vi "运维调试_总氮.vi"() -> ()   [LabVIEW 2016, in "斯坦道总氮.lvlib"]
uses:
  <vilib>/Utility/miscctls.llb/LVPointTypeDef.ctl
  <vilib>/Utility/config.llb/NI_LVConfig.lvlib
  <vilib>/ptbypt/NI_PtbyPt.lvlib
panel:
  in  "远程标样校准":enum16{"标液1", "标液2", "标液3", "标液4"}(ring)
  in  "远程校准量程":enum16{"低量程", "高量程"}(ring)
  out "固件版本号":string
  in  "定时设置":cluster{"启动":bool, "控制命令":T1, "测量参数":T2}(xcontrol)
  out "单位:":T3(ring)
  out "模块版本号":string
  in  "校准按钮":T4
  out "运行状态":T5 {"数据时间:" format="%<%y/%m/%d %H:%M:%S>T"; "仪器时间:" format="%<%y/%m/%d %H:%M:%S>T"}
  out "一级权限":bool
  out "二级权限":bool
  out "输入密码":u32
  out "布尔":bool
  in  "流程固件":bool
  in  "仪器参数设置":bool
  in  "量程参数读取":T6
  in  "模块启用":bool
  in  "串口设置":bool
  in  "公式一键写入":bool
  in  "流程路径":path=path "C:/Users/STD/Documents/斯坦道流程文件/流程.xml"
  in  "曲线模型":cluster{"X^2":dbl, "X":dbl, "B":dbl, "r^2":dbl}(xcontrol)
  out "字符串":string
  in  "质控参数设置":bool
  out "温度2":sgl
  out "温度1":sgl
  out "ADC":sgl
  in  "数组":string[](array[string])
  in  "量程切换阈值写入":bool
  in  "量程切换阈值读取":bool
  in  "参数下拉列表":enum16{"总磷", "总氮"}(ring)=enum."总氮"
  in  "量程下拉列表":enum16{"低量程", "高量程"}(ring)
  in  "测量模式下拉列表":enum16{"水样测量", "零点核查", "跨度核查", "标样核查", "加标回收"}(ring)
  in  "公式":cluster{"X^2":dbl, "X":dbl, "b":dbl}
  in  "写公式":bool
  in  "读公式":bool
  in  "返回":bool
  in  "设置":bool
  out "集成报警信息":string
  in  "停止":bool
  in  "手动启动":bool
  in  "单步测试":bool
  out "F3":sgl format="%#.6f"
  out "F2":sgl format="%#.6f"
  out "F1":sgl format="%#.6f"
  out "F0":sgl format="%#.6f"
  out "多列列表框":i32(listbox)
  # "参数设置"
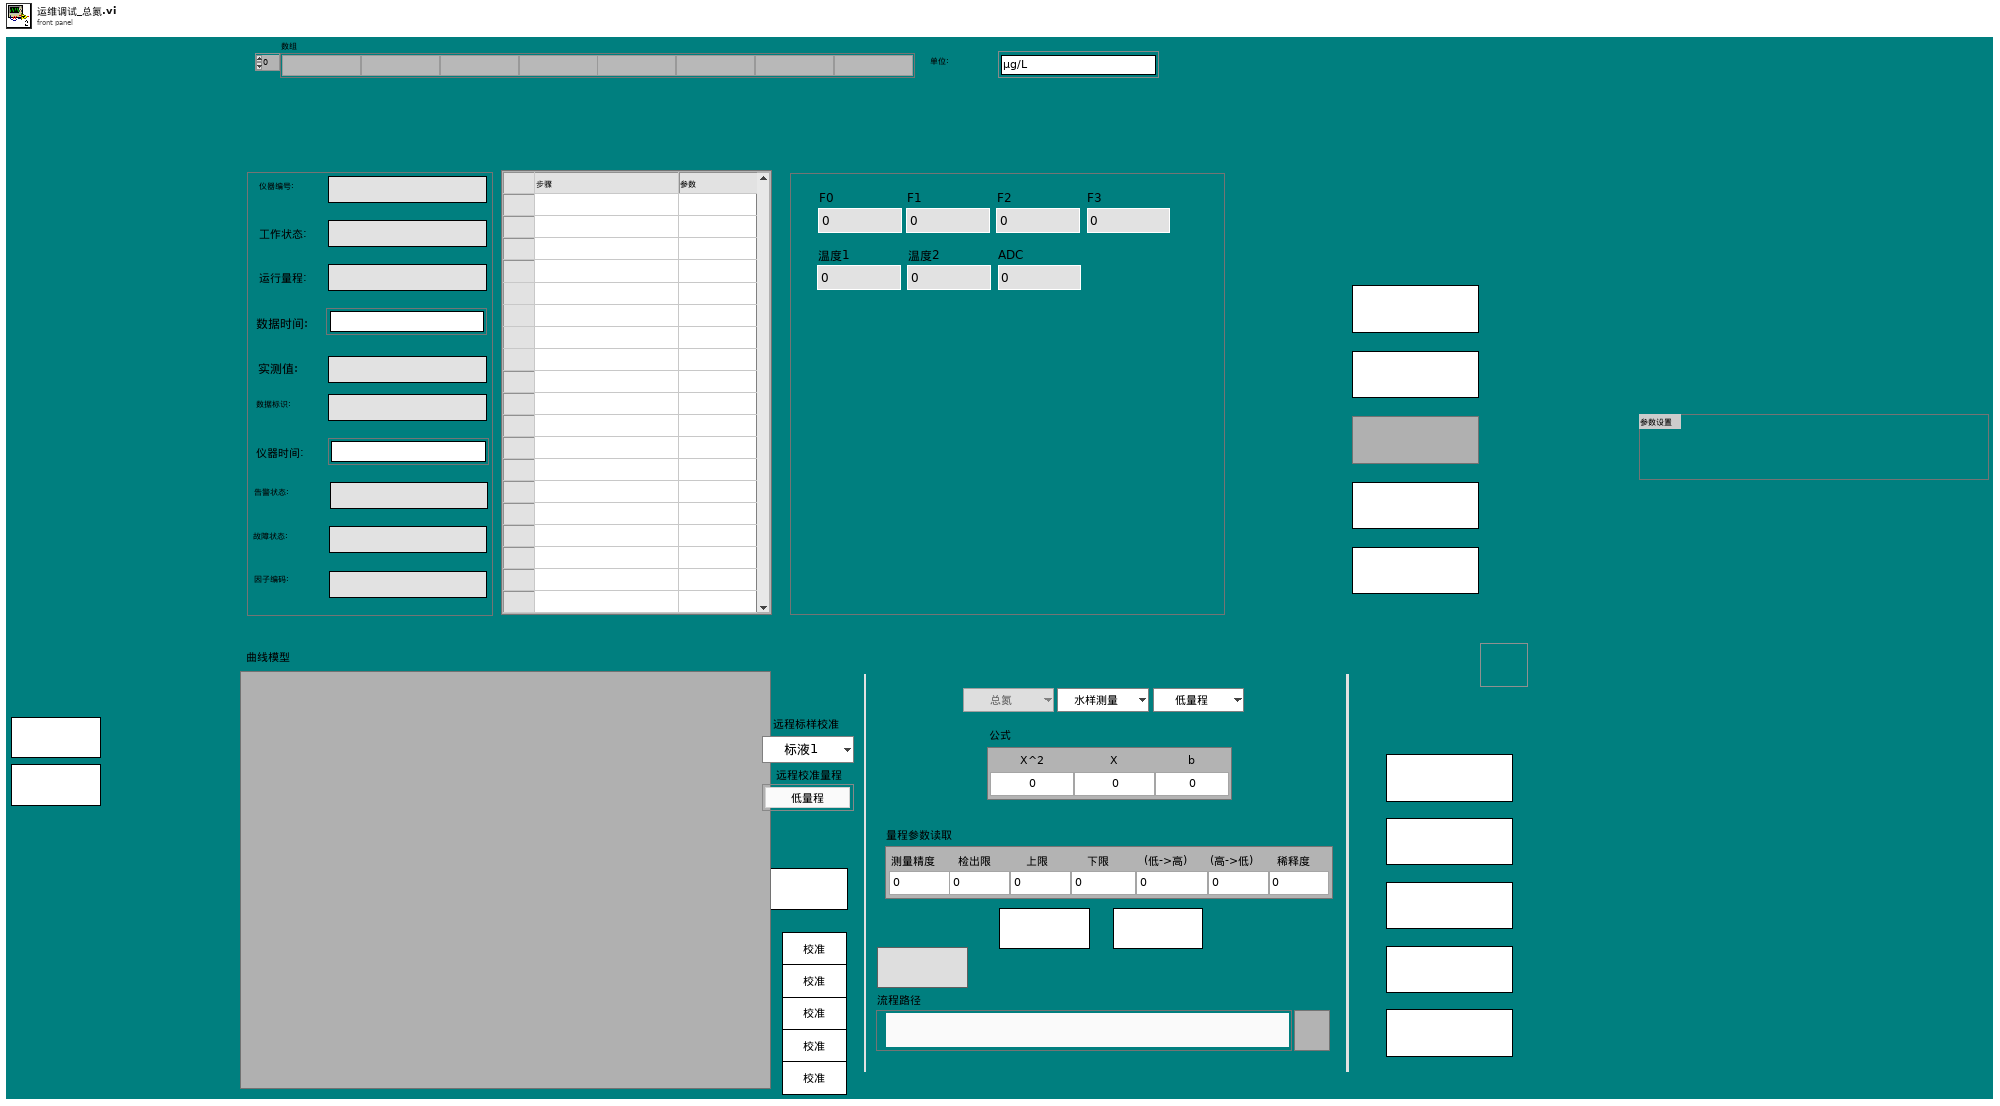
[diagram p1: front panel]
types:
  T1 = typedef "定时设置.xctl/国标控制命令.ctl" = enum16{"启动测量", "标样核查", "零点核查", "跨度核查", "空白测试", "平行样测试", "加标回收", "空白校准", "标样校准", "初始化（清洗）", "停止测试", "仪器重启", "校时", "模式设置", "测量间隔设置"}
  T2 = typedef "定时设置.xctl/测量参数.ctl" = u16
  T3 = enum16{"μg/L", "mg/L", "ppm", "mg/m3", "cm", "ppb", "μg/m3", "%", "nmol/mol", "μmol/mol", "MPN/L", "MPN/100ml", "ng/m3", "NTU", "无量纲", "mS/cm", "μS/cm", "℃", "mV", "cells/mL"}
  T4 = cluster{"校准1":bool, "校准2":bool, "校准3":bool, "校准4":bool, "校准5":bool}
  T5 = cluster{"仪器编号:":string, "工作状态:":string, "运行量程: ":string, "数据时间:":timestamp, "实测值:":string, "数据标识: ":string, "仪器时间:":timestamp, "告警状态: ":string, "故障状态:  ":string, "因子编码:":string}
  T6 = cluster{"测量精度":dbl, "检出限":dbl, "上限":dbl, "下限":dbl, "(低->高)":dbl, "(高->低)":dbl, "稀释度":dbl}
  T7 = typedef "LVPointTypeDef.ctl" = cluster{"Horizontal":i16, "Vertical":i16}
  T8 = cluster{"因子编码":u32, "单位":u16, "标样参考值":sgl, "水样数据时间":timestamp, "水样实测值":sgl, "水样数据标识":string, "标样数据时间":timestamp, "标样实测值":sgl, "标样数据标识":string, "空白数据时间":timestamp, "空白实测值":sgl, "空白数据标识":string, "零点核查数据时间":timestamp, "零点核查实测值":sgl, "零点核查数据标识":string, "跨度核查数据时间":timestamp, "跨度核查实测值":sgl, "跨度核查数据标识":string, "加标回收数据时间":timestamp, "加标回收实测值":sgl, "加标回收数据标识":string, "平行样数据时间":timestamp, "平行样实测值":sgl, "平行样数据标识":string, "F0":sgl, "F1":sgl, "F2":sgl, "F3":sgl, "F4":sgl, "F5":sgl, "F6":sgl, "F7":sgl, "温度":sgl, "湿度":sgl, "X值":sgl, "fidrange":u16}
  T9 = cluster{"系统时间":timestamp, "工作状态":enum16{"空闲", "水样测试", "标样核查", "零点核查", "跨度核查", "空白测试", "平行样测试", "加标回收", "空白校准", "标样校准", "初始化（清洗）"}, "测量模式":enum16{"待机", "连续模式", "周期模式", "定点模式", "受控模式", "手动模式"}, "告警代码":u16, "故障代码":u16, "日志代码":u16, "软件版本":u16, "F0":sgl, "F1":sgl, "F2":sgl, "F3":sgl, "T":sgl, "H":sgl, "id":u16, "flowid":u16, "量程":u16, "总磷控温温度1":sgl, "营养盐控温温度2":sgl, "ADC":sgl}
  T10 = enum16{"空闲", "水样测试", "标样核查", "零点核查", "跨度核查", "空白测试", "平行样测试", "加标回收", "空白校准", "标样校准", "初始化（清洗）"}
  T11 = cluster{"Major":u16, "Minor":u16, "Fix":u16, "Build":u16}
  T12 = typedef "NI_LVConfig.lvlib/Config Data RefNum.ctl" = refnum<k1>
  T13 = cluster{"时间源选择":enum16{"系统时间源", "仪器时间源"}, "外部时间源":timestamp}
  T14 = enum32{"Bad", "Idle", "Run top level", "Running"}
  T15 = enum8{"Enabled", "Disabled", "Disabled and Grayed Out"}
  T16 = cluster{"运行模式":enum16{"维护模式", "常规模式", "应急模式", "质控模式"}, "质控频次":enum16{"关闭", "每天", "星期一", "星期二", "星期三", "星期四", "星期五", "星期六", "星期日"}, "空白核查时间":u16, "跨度核查时间":u16, "24H周期设置":bool[]}
  T17 = cluster{"时间标识":timestamp, "设备":string, "日志信息":string, "备注":string}
  T18 = cluster{"参数":string, "报警内容":string, "报警分析":string}
  T19 = cluster{"启动模式":enum16{"跨度核查", "水样测量", "空白核查", "标样核查", "加标回收"}, "启动参数":u16, "量程":enum16{"低量程", "高量程"}}
  T20 = cluster{"时间标识":timestamp, "设备":string, "日志信息":string, "流程参数":string}
  T21 = typedef "LVRowAndColumnUnsignedTypeDef.ctl" = cluster{"Row":u32, "Column":u32}
  T22 = cluster{"参数下拉列表":enum16{"总磷", "总氮"}, "测量模式下拉列表":enum16{"水样测量", "零点核查", "跨度核查", "标样核查", "加标回收"}, "量程下拉列表":enum16{"低量程", "高量程"}}
  T23 = cluster{"站号":u16, "量程切换":enum32{"H", "L", "AUTO"}, "控制命令":enum16{"启动测量", "标样核查", "零点核查", "跨度核查", "空白测试", "平行样测试", "加标回收", "空白校准", "标样校准", "初始化（清洗）", "停止测试", "仪器重启", "校时", "模式设置", "测量间隔设置"}, "模式设置":enum16{"待机", "连续模式", "周期模式", "定点模式", "受控模式", "手动模式"}, "测量间隔":u16}
  T24 = cluster{"水样测试量程模式":enum16{"H", "L", "AUTO"}, "空白核查量程模式":enum16{"H", "L", "AUTO"}, "跨度核查量程模式":enum16{"H", "L", "AUTO"}, "加标回收量程模式":enum16{"H", "L", "AUTO"}}
  T25 = cluster{"跨度值":dbl, "零点标准液浓度":dbl, "跨度标准液浓度":dbl, "标准液标准浓度":dbl}
  T26 = cluster{"确定":bool, "跨度值":dbl, "零点标准液浓度":dbl, "跨度标准液浓度":dbl, "标准液标准浓度":dbl}
  T27 = cluster{"测量量程":dbl, "测量精度":dbl, "测量间隔":dbl, "消解温度":dbl, "消解时长":dbl, "空白校准时间":timestamp, "曲线截距":dbl, "曲线斜率":dbl, "测量检出限":dbl, "测量信号值":dbl, "线性相关系数":dbl, "二次多项式系数":dbl, "标样校准时间":timestamp, "稀释倍数":dbl, "三项式系数":dbl, "空白标定系数":dbl, "量程系数":dbl, "F0/ORPA":dbl, "F1/ORPB":dbl, "F2/ORPK":dbl, "F3":dbl, "F4":dbl, "F5":dbl, "F6":dbl, "F7":dbl, "X0/滴定数":dbl, "量程":dbl}
  T28 = cluster{"确定":bool, "测量量程":dbl, "测量精度":dbl, "测量间隔":dbl, "消解温度":dbl, "消解时长":dbl, "空白校准时间":timestamp, "曲线截距":dbl, "曲线斜率":dbl, "测量检出限":dbl, "测量信号值":dbl, "线性相关系数":dbl, "二次多项式系数":dbl, "标样校准时间":timestamp, "稀释倍数":dbl, "三项式系数":dbl, "空白标定系数":dbl, "量程系数":dbl, "F0/ORPA":dbl, "F1/ORPB":dbl, "F2/ORPK":dbl, "F3":dbl, "F4":dbl, "F5":dbl, "F6":dbl, "F7":dbl, "X0/滴定数":dbl, "量程":dbl}
  T29 = cluster{"标液浓度1":dbl, "标液浓度2":dbl, "标液浓度3":dbl, "标液浓度4":dbl, "标液浓度5":dbl}
  T30 = cluster{"测量精度":u16, "检出限":dbl, "上限":dbl, "下限":dbl, "阈值（低->高）":dbl, "阈值（高->低）":dbl, "稀释度":dbl}
  T31 = enum16{"Left Button", "Center Button", "Right Button", "Window Close"}
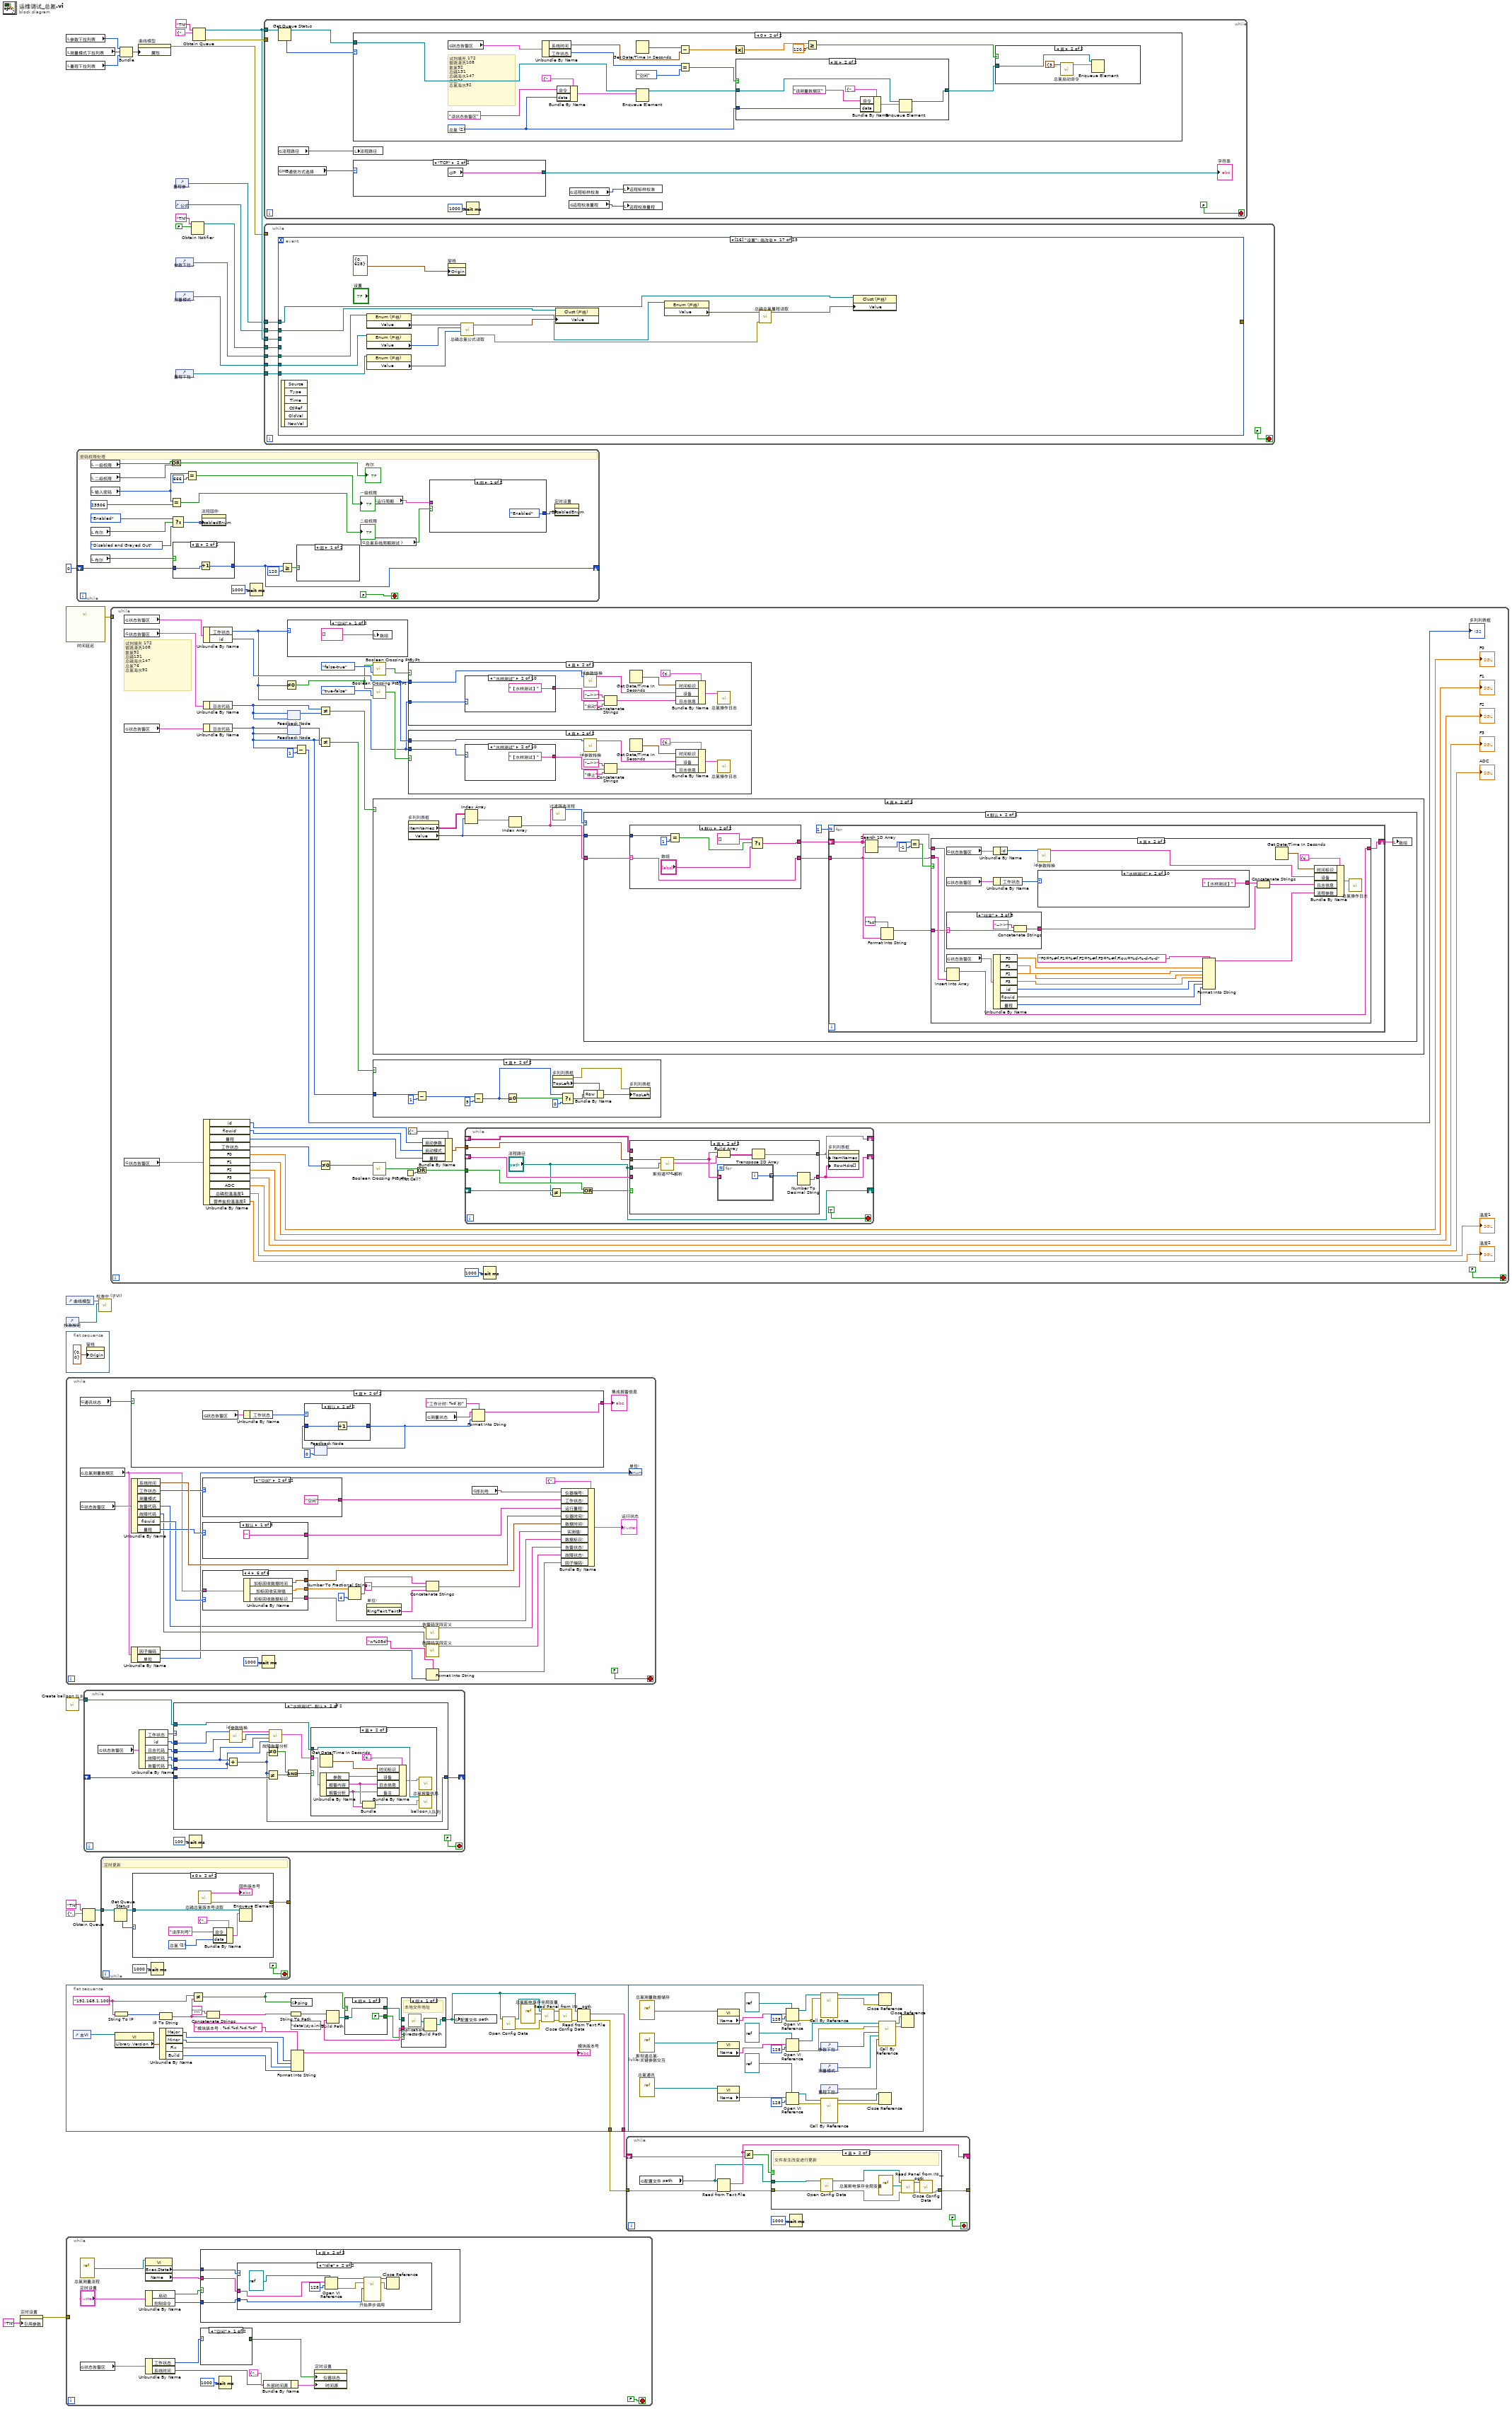
[diagram p0: block diagram]
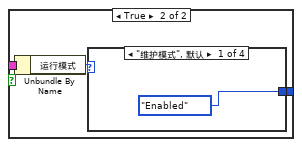
[diagram p5: hidden frame]
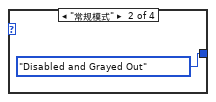
[diagram p6: hidden frame]
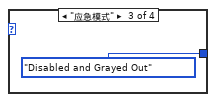
[diagram p7: hidden frame]
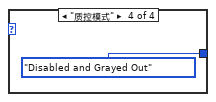
[diagram p8: hidden frame]
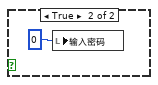
[diagram p9: hidden frame]
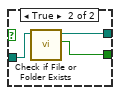
[diagram p11: hidden frame]
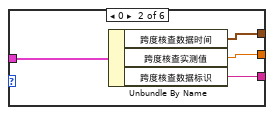
[diagram p15: hidden frame]
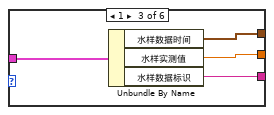
[diagram p16: hidden frame]
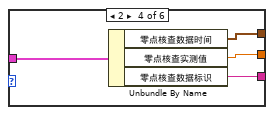
[diagram p17: hidden frame]
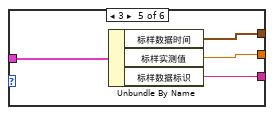
[diagram p18: hidden frame]
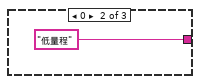
[diagram p19: hidden frame]
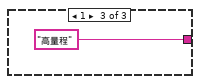
[diagram p20: hidden frame]
diagram:
  n1 = property on="定时设置" class="定时设置 (严格)"("引用参数"="TN") -> (error out=w1:errorcluster)  [unwired: 2 in, 1 out]
  n2 = local read "参数下拉列表"() -> (w12:enum16{"总磷", "总氮"})
  n3 = local read "测量模式下拉列表"() -> (w11:enum16{"水样测量", "零点核查", "跨度核查", "标样核查", "加标回收"})
  n4 = local read "量程下拉列表"() -> (w10:enum16{"低量程", "高量程"})
  n5 = call "时间延迟"() -> ("error out"=w21:errorcluster)  [unwired: 11 in]
  n6 = control-ref of="曲线模型"() -> (w6:refnum<vi>)
  n7 = control-ref of="校准按钮"() -> (w5:refnum<vi>)
  n8 = flat-sequence {
    frame #0 {
      n9 = property on="窗格" class="Pane"("Origin"=T7 {"Horizontal"=0, "Vertical"=0} ("原点")) -> ()  [unwired: 2 in, 2 out]
    }
  }
  n10 = while {
    stop <- FALSE stop-if-true
    n11 = global read "VAR总氮全局变量.vi" "通讯状态"() -> (w59:bool)
    n12 = global read "VAR总氮全局变量.vi" "总氮测量数据区"() -> (w48:T8)
    n13 = global read "VAR总氮全局变量.vi" "状态告警区"() -> (w51:T9)
    n14 = case shown="真" w59 {
      tunnel: ["通讯异常" ("集成报警信息") w102] -> w58
      frame False {
      }
      frame True {
        n15 = global read "VAR总氮全局变量.vi" "状态告警区"() -> (w108:T9)
        n16 = Unbundle By Name(w108) -> ("工作状态"=w107:T10)
        n17 = feedback #1(0) -> (w105:i32)
        n18 = case shown="默认" w107 {
          tunnel: w105 -> [_ w110]
          tunnel: [_ w109] -> w103
          frame "空闲" {
          }
          frame Default {
            n19 = Increment(x=w110) -> (x+1=w109:i32)
          }
        }
        n20 = feedback-in #1(w103) -> ()
        n21 = global read "VAR总氮全局变量.vi" "测量状态"() -> (w101:string)
        n22 = Format Into String(format string="工作计时: %d 秒" ("格式字符串"), initial string=w101, w103) -> (resulting string=w102:string)  [unwired: 1 in, 1 out]
      }
    }
    "集成报警信息" <- w58
    n23 = Unbundle By Name(w51) -> ("系统时间"=w57:timestamp, "工作状态"=w49:T10, "告警代码"=w34:u16, "故障代码"=w32:u16, "flowid"=w47:u16, "量程"=w55:u16)  [unwired: 1 out]
    n24 = Unbundle By Name(w48) -> ("因子编码"=w52:u32, "单位"=→"单位:":u16)
    n25 = case shown="\"空闲\"" w49 {
      selector: w49 -> [w85 _ _ _ _ _ _ _ _ _ _ _]
      tunnel: [w86 "空闲" ("工作状态") "水样测量" ("工作状态") "标样核查" ("工作状态") "零点核查" ("工作状态") "跨度核查" ("工作状态") "空白测试" ("工作状态") "平行样测试" ("工作状态") "加标回收" ("工作状态") "空白校准" ("工作状态") "标样校准" ("工作状态") "初始化" ("工作状态")] -> w56
      frame Default {
        n26 = Format Into String(format string="%d" ("格式字符串"), initial string="未知" ("工作状态"), w85) -> (resulting string=w86:string)  [unwired: 1 in, 1 out]
      }
      frame "空闲" {
      }
      frame "水样测试" {
      }
      frame "标样核查" {
      }
      frame "零点核查" {
      }
      frame "跨度核查" {
      }
      frame "空白测试" {
      }
      frame "平行样测试" {
      }
      frame "加标回收" {
      }
      frame "空白校准" {
      }
      frame "标样校准" {
      }
      frame "初始化（清洗）" {
      }
    }
    n27 = case shown="默认" w55 {
      tunnel: ["" ("字符串") "低量程" ("字符串") "高量程" ("字符串")] -> w54
      frame Default {
      }
      frame 0 {
      }
      frame 1 {
      }
    }
    n28 = case shown="4" w47 {
      tunnel: [_ w65 w69 w73 w77 w81] -> w43
      tunnel: [_ w63 w68 w72 w76 w80] -> w39
      tunnel: [_ w62 w67 w71 w75 w79] -> w36
      tunnel: w48 -> [_ w64 w66 w70 w74 w78]
      frame Default {
      }
      frame 0 {
        n29 = Unbundle By Name(w64) -> ("跨度核查数据时间"=w65:timestamp, "跨度核查实测值"=w63:sgl, "跨度核查数据标识"=w62:string)
      }
      frame 1 {
        n30 = Unbundle By Name(w66) -> ("水样数据时间"=w69:timestamp, "水样实测值"=w68:sgl, "水样数据标识"=w67:string)
      }
      frame 2 {
        n31 = Unbundle By Name(w70) -> ("零点核查数据时间"=w73:timestamp, "零点核查实测值"=w72:sgl, "零点核查数据标识"=w71:string)
      }
      frame 3 {
        n32 = Unbundle By Name(w74) -> ("标样数据时间"=w77:timestamp, "标样实测值"=w76:sgl, "标样数据标识"=w75:string)
      }
      frame 4 {
        n33 = Unbundle By Name(w78) -> ("加标回收数据时间"=w81:timestamp, "加标回收实测值"=w80:sgl, "加标回收数据标识"=w79:string)
      }
    }
    n34 = Wait (ms)(milliseconds to wait=u32 1000 ("等待时间（毫秒）")) -> ()  [unwired: 1 out]
    n35 = Number To Fractional String(number=w39, precision (6)=i16 4 ("精度(6)")) -> (F-format string=w38:string)  [unwired: 2 in]
    n36 = property on="单位:" class="Enum (严格)"() -> ("RingText.Text"=w40:string)  [unwired: 2 in, 2 out]
    n37 = Concatenate Strings(w38, " " ("字符串"), w40) -> (w37:string)
    n38 = call "告警码字段定义.vi"("告警代码"=w34) -> ("字符串"=w33:string)  [unwired: 8 in, 2 out]
    n39 = call "故障码字段定义.vi"("故障代码"=w32) -> ("字符串"=w31:string)  [unwired: 10 in]
    n40 = Format Into String(format string="w%05d" ("格式字符串"), w52) -> (resulting string=w35:string)  [unwired: 2 in, 1 out]
    n41 = global read "VAR总氮全局变量.vi" "序列号"() -> (w50:string)
    n42 = Bundle By Name(cluster=T5 {"仪器编号:"="", "工作状态:"="", "运行量程: "="", "数据时间:"=timestamp(0 s since 1904-01-01), "实测值:"="", "数据标识: "="", "仪器时间:"=timestamp(0 s since 1904-01-01), "告警状态: "="", "故障状态:  "="", "因子编码:"=""} ("运行状态"), "仪器编号:"=w50, "工作状态:"=w56, "运行量程:"=w54, "仪器时间:"=w57, "数据时间:"=w43, "实测值:"=w37, "数据标识:"=w36, "告警状态:"=w33, "故障状态:"=w31, "因子编码:"=w35) -> (→"运行状态":T5)
  }
  n43 = call "Create balloon 队列.vi"() -> ("队列输出"=w3:refnum<queue>)  [unwired: 11 in]
  n44 = flat-sequence {
    tunnel: [w120] -> w4
    tunnel: [w119] -> w7
    frame #0 {
      w133 = "data\\sys.ini" ("名称或相对路径")
      w125 = "192.168.1.100" ("名称")
      n45 = control-ref of="本VI"() -> (w118:refnum<vi>)
      n46 = String To IP(1:w125) -> (0:w132:u32)
      n47 = property class="VI"(reference=w118) -> ("Library.Version"=w117:T11)  [unwired: 1 in, 2 out]
      n48 = IP To String(2:w132) -> (0:w129:string)  [unwired: 1 in]
      n49 = Unbundle By Name(w117) -> ("Major"=w115:u16, "Minor"=w114:u16, "Fix"=w113:u16, "Build"=w112:u16)
      n50 = Not Equal?(x=w125, y=w129) -> (x != y?=w123:bool)
      n51 = Concatenate Strings("\\\\" ("字符串"), w129) -> (w130:string)
      n52 = String To Path(string=w130) -> (path=w124:path)
      n53 = global write "VAR总氮全局变量.vi" "ping"(w123) -> ()
      n54 = Format Into String(format string="模块版本号：%d.%d.%d.%d" ("格式字符串"), w115, w114, w113, w112) -> (resulting string=→"模块版本号":string)  [unwired: 2 in, 1 out]
      n55 = Build Path(base path=w124, name or relative path=w133) -> (appended path=w128:path)
      n56 = case shown="假" w123 {
        tunnel: w128 -> [w139 w143]
        tunnel: [w139 w142] -> w127
        tunnel: [FALSE w141] -> w126
        frame False {
        }
        frame True {
          n57 = call <vilib>:"Check if File or Folder Exists.vi"("path"=w143) -> ("file or folder exists?"=w141:bool, "dup path"=w142:path)  [unwired: 8 in, 1 out]
        }
      }
      n58 = case shown="假" w126 {
        tunnel: w127 -> [_ w147]
        tunnel: [w145 w147] -> w122
        tunnel: w133 -> [w144 _]
        frame False {
          # "本地文件地址"
          n59 = call <vilib>:"Application Directory.vi"() -> ("Application Directory"=w146:path)
          n60 = Build Path(base path=w146, name or relative path=w144) -> (appended path=w145:path)
        }
        frame True {
          # "网络共享地址"
        }
      }
      n61 = global write "VAR总氮全局变量.vi" "配置文件 path"(w122) -> ()
      n62 = call <vilib>:"Open Config Data.vi"("configuration file path"=w122) -> ("error out"=w135:errorcluster, "refnum"=w138:T12)  [unwired: 8 in, 1 out]
      n63 = vi-ref "总氮断电保存全局变量.vi"() -> (w137:refnum<vi>)
      n64 = call <userlib>:"Read Panel from INI__ogtk.vi"("error in (no error)"=w135, "VI ref"=w137, "refnum"=w138) -> ("error out"=w134:errorcluster, "refnum out"=w136:T12)  [unwired: 7 in]
      n65 = call <vilib>:"Close Config Data.vi"("error in (no error)"=w134, "refnum"=w136) -> ("error out"=w121:errorcluster)  [unwired: 8 in, 1 out]
      n66 = Read from Text File(file (use dialog)=w122, error in=w121) -> (text=w119:string, error out=w120:errorcluster)  [unwired: 2 in, 2 out]
    }
    frame #1 {
      n67 = vi-ref "总氮测量数据储存.vi"() -> (w166:refnum<vi>)
      n68 = vi-ref "斯坦道总氮.lvlib:关键参数交互.vi"() -> (w151:refnum<vi>)
      n69 = vi-ref "总氮通讯.vi"() -> (w174:refnum<vi>)
      n70 = property class="VI"(reference=w166) -> ("Name"=w159:string)  [unwired: 1 in, 2 out]
      n71 = property class="VI"(reference=w151) -> ("Name"=w158:string)  [unwired: 1 in, 2 out]
      n72 = property class="VI"(reference=w174) -> ("Name"=w173:string)  [unwired: 1 in, 2 out]
      n73 = Open VI Reference(type specifier VI Refnum (for type only)=refnum<vi> refnum, vi path=w159, options=128 ("选项")) -> (vi reference=w161:refnum<vi>, error out=w163:errorcluster)  [unwired: 3 in]
      n74 = Open VI Reference(type specifier VI Refnum (for type only)=refnum<vi> refnum, vi path=w158, options=128 ("选项")) -> (vi reference=w156:refnum<vi>, error out=w154:errorcluster)  [unwired: 3 in]
      n75 = Open VI Reference(type specifier VI Refnum (for type only)=refnum<vi> refnum, vi path=w173, options=128 ("选项")) -> (vi reference=w171:refnum<vi>, error out=w169:errorcluster)  [unwired: 3 in]
      n76 = call-by-ref "?"(reference=w161, error in=w163) -> (reference out=w165:refnum<vi>, error out=w164:errorcluster)  [unwired: 12 in]
      n77 = control-ref of="参数下拉列表"() -> (w150:refnum<vi>)
      n78 = control-ref of="测量模式下拉列表"() -> (w149:refnum<vi>)
      n79 = control-ref of="量程下拉列表"() -> (w148:refnum<vi>)
      n80 = call-by-ref "?"(reference=w171, error in=w169) -> (reference out=w167:refnum<vi>, error out=w168:errorcluster)  [unwired: 12 in]
      n81 = Close Reference(reference=w165, error in (no error)=w164) -> ()  [unwired: 1 out]
      n82 = call-by-ref "?"(reference=w156, error in=w154, "量程下拉列表"=w148, "测量模式下拉列表"=w149, "测量参数"=w150) -> (reference out=w152:refnum<vi>, error out=w153:errorcluster)  [unwired: 9 in]
      n83 = Close Reference(reference=w167, error in (no error)=w168) -> ()  [unwired: 1 out]
      n84 = Close Reference(reference=w152, error in (no error)=w153) -> ()  [unwired: 1 out]
    }
  }
  n85 = while {
    tunnel: w1 -> [_]
    stop <- FALSE stop-if-true
    n86 = vi-ref "总氮测量流程.vi"() -> (w186:refnum<vi>)
    n87 = global read "VAR总氮全局变量.vi" "状态告警区"() -> (w180:T9)
    n88 = property class="VI"(reference=w186) -> ("Exec.State"=w184:T14, "Name"=w185:string)  [unwired: 1 in, 2 out]
    n89 = Unbundle By Name("定时设置") -> ("启动"=w181:bool, "控制命令"=w182:T1)
    n90 = Unbundle By Name(w180) -> ("工作状态"=w179:T10, "系统时间"=w175:timestamp)
    n91 = case shown="真" w181 {
      tunnel: w185 -> [_ w192]
      tunnel: w182 -> [_ w191]
      tunnel: w184 -> [_ w190]
      frame False {
      }
      frame True {
        n92 = case shown="\"Idle\"" w190 {
          tunnel: w192 -> [_ w196]
          tunnel: w191 -> [_ w194]
          frame "Bad", Default {
          }
          frame "Idle" {
            n93 = Open VI Reference(type specifier VI Refnum (for type only)=refnum<vi> refnum, vi path=w196, options=128 ("选项")) -> (vi reference=w197:refnum<vi>, error out=w198:errorcluster)  [unwired: 3 in]
            n94 = call-by-ref "开始异步调用"(reference=w197, error in=w198, "控制命令"=w194) -> (reference out=w199:refnum<vi>, error out=w200:errorcluster)  [unwired: 11 in]
            n95 = Close Reference(reference=w199, error in (no error)=w200) -> ()  [unwired: 1 out]
          }
        }
      }
    }
    n96 = case shown="\"空闲\"" w179 {
      tunnel: [_ TRUE] -> w178
      frame "空闲" {
      }
      frame "水样测试", Default {
      }
    }
    n97 = Wait (ms)(milliseconds to wait=u32 1000 ("等待时间（毫秒）")) -> ()  [unwired: 1 out]
    n98 = Bundle By Name(cluster=T13 {"时间源选择"=enum."仪器时间源", "外部时间源"=timestamp(0 s since 1904-01-01)} ("时间源"), "外部时间源"=w175) -> (w176:T13)
    n99 = property on="定时设置" class="定时设置 (严格)"("仪器状态"=w178, "时间源"=w176) -> ()  [unwired: 2 in, 2 out]
  }
  n100 = while {
    shift-right: [w210] -> _
    shift-left: u32 0 ("等待时间（毫秒）") -> [w211]
    stop <- FALSE stop-if-true
    # "密码权限处理"
    n101 = local read "一级权限"() -> (w214:bool)
    n102 = local read "二级权限"() -> (w215:bool)
    n103 = local read "输入密码"() -> (w218:u32)
    n104 = local read "布尔"() -> (w207:bool)
    n105 = local read "布尔"() -> (w212:bool)
    n106 = Or(x=w214, y=w215) -> (x .or. y?=→"布尔":bool)
    n107 = Equal?(x=w218, y=u32 23506) -> (x = y?=→"二级权限":bool)
    n108 = Select(t=T15."Enabled" ("禁用"), s=w207, f=T15."Disabled and Grayed Out") -> (s? t:f=w205:T15)
    n109 = case shown="真" w212 {
      tunnel: w211 -> [_ w233]
      tunnel: [_ w232] -> w210
      frame False {
      }
      frame True {
        n110 = Increment(x=w233) -> (x+1=w232:u32)
      }
    }
    n111 = Equal?(x=w218, y=u32 666) -> (x = y?=→"一级权限":bool)
    n112 = property on="流程固件" class="Bool"("DisabledEnum"=w205) -> ()  [unwired: 2 in, 2 out]
    n113 = Wait (ms)(milliseconds to wait=u32 1000 ("等待时间（毫秒）")) -> ()  [unwired: 1 out]
    n114 = Greater Or Equal?(x=w210, y=u32 120) -> (x >= y?=w208:bool)
    n115 = case shown="假" w208 {
      frame False {
      }
      frame True {
        n116 = local write "输入密码"(u32 0 ("输入密码")) -> ()
      }
    }
    n117 = global read "总氮断电保存全局变量.vi" "总氮系统周期测试？"() -> (w202:bool)
    n118 = global read "总氮断电保存全局变量.vi" "运行周期"() -> (w203:T16)
    n119 = case shown="假" w202 {
      tunnel: w203 -> [_ w226]
      tunnel: [T15."Enabled" ("禁用") w224] -> w201
      frame False {
      }
      frame True {
        n120 = Unbundle By Name(w226) -> ("运行模式"=w225:enum16{"维护模式", "常规模式", "应急模式", "质控模式"})
        n121 = case shown="\"维护模式\", 默认" w225 {
          tunnel: [T15."Enabled" ("禁用") T15."Disabled and Grayed Out" ("禁用") T15."Disabled and Grayed Out" ("禁用") T15."Disabled and Grayed Out" ("禁用")] -> w224
          frame "维护模式", Default {
          }
          frame "常规模式" {
          }
          frame "应急模式" {
          }
          frame "质控模式" {
          }
        }
      }
    }
    n122 = property on="定时设置" class="定时设置 (严格)"("DisabledEnum"=w201) -> ()  [unwired: 2 in, 2 out]
  }
  n123 = Obtain Queue(name (unnamed)="TN" ("名称（未命名）"), element data type=cluster{"命令":string, "data":variant} {"命令"="", "data"=variant}) -> (queue out=w18:refnum<queue>)  [unwired: 3 in, 2 out]
  n124 = while {
    tunnel: w3 -> [w240]
    shift-right: [w236] -> _
    shift-left: _ -> [w237]
    stop <- FALSE stop-if-true
    n125 = global read "VAR总氮全局变量.vi" "状态告警区"() -> (w234:T9)
    n126 = Unbundle By Name(w234) -> ("工作状态"=w235:T10, "id"=w242:u16, "日志代码"=w241:u16, "故障代码"=w239:u16, "告警代码"=w238:u16)
    n127 = case shown="\"水样测试\", 默认" w235 {
      tunnel: w242 -> [_ w257]
      tunnel: w241 -> [_ w256]
      tunnel: w240 -> [_ w253]
      tunnel: w239 -> [_ w252]
      tunnel: w238 -> [_ w251]
      tunnel: w237 -> [w245 w250]
      tunnel: [w245 w249] -> w236
      frame "空闲" {
      }
      frame "水样测试", Default {
        n128 = Add(x=w252, y=w251) -> (x+y=w249:u16)
        n129 = call "id参数转换.vi"("id"=w257) -> ("table输出"=w254:string)  [unwired: 10 in]
        n130 = Not Equal To 0?(x=w249) -> (x != 0?=w248:bool)
        n131 = Not Equal?(x=w249, y=w250) -> (x != y?=w247:bool)
        n132 = call "故障告警分析.vi"("告警代码"=w251, "故障代码"=w252, "运行步序"=w256, "参数"=w254) -> ("报警内容"=w255:T18)  [unwired: 6 in, 1 out]
        n133 = And(x=w248, y=w247) -> (x .and. y?=w246:bool)
        n134 = case shown="真" w246 {
          tunnel: w255 -> [_ w266]
          tunnel: w253 -> [_ w265]
          frame False {
          }
          frame True {
            n135 = Get Date/Time In Seconds() -> (seconds since 1Jan1904=w264:timestamp)
            n136 = Unbundle By Name(w266) -> ("参数"=w261:string, "报警内容"=w260:string, "报警分析"=w259:string)
            n137 = Bundle("报警内容"=w260, "报警分析"=w259) -> (w258:cluster{"报警内容":string, "报警分析":string})  [unwired: 1 in]
            n138 = Bundle By Name(cluster=T17 {"时间标识"=timestamp(0 s since 1904-01-01), "设备"="", "日志信息"="", "备注"=""} ("data in"), "时间标识"=w264, "设备"=w261, "日志信息"=w260, "备注"=w259) -> (w263:T17)
            n139 = call "总氮报警信息.vi"("data in"=w263) -> ()  [unwired: 10 in, 1 out]
            n140 = call "balloon入队列.vi"("报警内容"=w258, "队列"=w265) -> ()  [unwired: 9 in, 1 out]
          }
        }
      }
    }
    n141 = Wait (ms)(milliseconds to wait=u32 100) -> ()  [unwired: 1 out]
  }
  n142 = call "校准中 (子VI).vi"("曲线模型"=w6, "校准按钮"=w5) -> ()  [unwired: 9 in]
  n143 = while {
    tunnel: w18 -> [w271]
    tunnel: [w269] -> _
    stop <- FALSE stop-if-true
    # "定时更新"
    n144 = Get Queue Status(queue=w271) -> (queue out=w268:refnum<queue>, # elements in queue=w267:i32)  [unwired: 2 in, 6 out]
    n145 = case shown="0" w267 {
      tunnel: [_ w275] -> w269
      tunnel: w268 -> [_ w274]
      frame Default {
      }
      frame 0 {
        w277 = u16 2 items=["总磷"=1, "总氮"=2, "氨氮"=3] ("站号")
        n146 = call "总磷总氮版本号读取.vi"() -> ("error out"=w275:errorcluster, "固件版本号"=→"固件版本号":string)  [unwired: 10 in]
        n147 = Bundle By Name(cluster=cluster{"命令":string, "data":variant} {"命令"="", "data"=variant} ("元素"), "命令"="读序列号", "data"=w277) -> (w276:cluster{"命令":string, "data":variant})
        n148 = Enqueue Element(queue=w274, element=w276) -> ()  [unwired: 2 in, 3 out]
      }
    }
    n149 = Wait (ms)(milliseconds to wait=u32 1000 ("等待时间（毫秒）")) -> ()  [unwired: 1 out]
  }
  n150 = while {
    tunnel: w21 -> [_]
    stop <- FALSE stop-if-true
    # "试剂填充 172 \n管路清洗108\n氨氮92\n总磷131\n总磷海水147\n总氮76\n总氮海水92"
    n151 = global read "VAR总氮全局变量.vi" "状态告警区"() -> (w300:T9)
    n152 = global read "VAR总氮全局变量.vi" "状态告警区"() -> (w298:T9)
    n153 = global read "VAR总氮全局变量.vi" "状态告警区"() -> (w302:T9)
    n154 = global read "VAR总氮全局变量.vi" "状态告警区"() -> (w310:T9)
    n155 = Unbundle By Name(w300) -> ("工作状态"=w280:T10, "id"=w284:u16)
    n156 = Unbundle By Name(w298) -> ("日志代码"=w297:u16)
    n157 = Unbundle By Name(w302) -> ("日志代码"=w294:u16)
    n158 = Unbundle By Name(w310) -> ("id"=w307:u16, "flowid"=w309:u16, "量程"=w308:u16, "工作状态"=w288:T10, "F0"=→"F0":sgl, "F1"=→"F1":sgl, "F2"=→"F2":sgl, "F3"=→"F3":sgl, "ADC"=→"ADC":sgl, "总磷控温温度1"=→"温度1":sgl, "营养盐控温温度2"=→"温度2":sgl)
    n159 = Not Equal To 0?(x=w280) -> (x != 0?=w282:bool)
    n160 = case shown="\"空闲\"" w280 {
      frame "空闲" {
        n161 = local write "数组"(string[] [] ("数组")) -> ()
      }
      frame "水样测试", Default {
      }
    }
    n162 = feedback #2(w297) -> (w299:u16)
    n163 = feedback-in #2(w297) -> ()
    n164 = feedback-in #3(w294) -> ()
    n165 = feedback #3(w294) -> (w315:u16)
    n166 = Subtract(x=w294, y=1) -> (x-y=→"多列列表框":i32)
    n167 = Not Equal?(x=w297, y=w299) -> (x != y?=w296:bool)
    n168 = Not Equal?(x=w294, y=w315) -> (x != y?=w314:bool)
    n169 = Not Equal To 0?(x=w288) -> (x != 0?=w312:bool)
    n170 = call <vilib>:"Boolean Crossing PtByPt.vi"("direction"=enum16{"either", "false-true", "true-false"}."false-true", "input"=w282) -> ("crossing"=w286:bool)  [unwired: 1 in]
    n171 = call <vilib>:"Boolean Crossing PtByPt.vi"("direction"=enum16{"either", "false-true", "true-false"}."true-false", "input"=w282) -> ("crossing"=w281:bool)  [unwired: 1 in]
    n172 = case shown="真" w296 {
      frame False {
      }
      frame True {
        n173 = property on="多列列表框" class="MCListbox (严格)"() -> ("ItemNames"=w361:string[][], "Value"=w357:i32)  [unwired: 2 in, 2 out]
        n174 = Index Array(array=w361, index (row)=w357) -> (element=w360:string[])  [unwired: 1 in]
        n175 = Index Array(array=w360) -> (element=w359:string)  [unwired: 1 in]
        n176 = call "过滤筛选流程.vi"("字符串"=w359) -> ("匹配后偏移量"=w358:i32)  [unwired: 10 in]
        n177 = case shown="默认" w358 {
          tunnel: w359 -> [_ w363]
          tunnel: w357 -> [_ w362]
          frame -1 {
          }
          frame Default {
            n178 = case shown="默认" w363 {
              selector: w363 -> [w369 w376]
              tunnel: [w369 w376] -> w365
              tunnel: [string[] [] ("数组") w371] -> w364
              tunnel: w362 -> [_ w375]
              frame "读数" {
              }
              frame Default {
                n179 = Equal?(x=w375, y=1) -> (x = y?=w373:bool)
                n180 = Select(t=string[] [], s=w373, f="数组") -> (s? t:f=w371:string[])
              }
            }
            n181 = for {
              N: 1 -> [_]
              tunnel: w365 -> [w378]
              shift-right: [w377] -> w366
              shift-left: w364 -> [w379]
              n182 = Search 1D Array(1D array=w379, element=w378) -> (index of element=w382:i32)  [unwired: 1 in]
              n183 = Format Into String(format string="%s" ("格式字符串"), w378) -> (resulting string=w383:string)  [unwired: 2 in, 1 out]
              n184 = Equal?(x=w382, y=-1) -> (x = y?=w380:bool)
              n185 = case shown="真" w380 {
                tunnel: w383 -> [_ w393]
                tunnel: w379 -> [w385 w397]
                tunnel: w378 -> [_ w396]
                tunnel: [w385 w395] -> w377
                frame False {
                }
                frame True {
                  n186 = global read "VAR总氮全局变量.vi" "状态告警区"() -> (w410:T9)
                  n187 = global read "VAR总氮全局变量.vi" "状态告警区"() -> (w392:T9)
                  n188 = case shown="\"结束\"" w393 {
                    selector: w393 -> [w420 w423 w426]
                    tunnel: [w420 w422 w425] -> w389
                    frame Default {
                    }
                    frame "初始化" {
                      n189 = Concatenate Strings("-->>" ("字符串"), w423) -> (w422:string)
                    }
                    frame "结束" {
                      n190 = Concatenate Strings("-->>" ("字符串"), w426) -> (w425:string)
                    }
                  }
                  n191 = global read "VAR总氮全局变量.vi" "状态告警区"() -> (w407:T9)
                  n192 = Insert Into Array(array=w397, new element=w396) -> (w395:string[])  [unwired: 1 in]
                  n193 = Unbundle By Name(w410) -> ("id"=w387:u16)
                  n194 = Unbundle By Name(w392) -> ("工作状态"=w391:T10)
                  n195 = Unbundle By Name(w407) -> ("F0"=w404:sgl, "F1"=w403:sgl, "F2"=w402:sgl, "F3"=w401:sgl, "id"=w400:u16, "flowid"=w399:u16, "量程"=w398:u16)
                  n196 = call "id参数转换.vi"("id"=w387) -> ("table输出"=w386:string)  [unwired: 10 in]
                  n197 = case shown="\"水样测试\"" w391 {
                    tunnel: [_ "【水样测试】" ("字符串") "【标样核查】" ("字符串") "【零点核查】" ("字符串") "【跨度核查】" ("字符串") "【空白测试】" ("字符串") "【平行样测试】" ("字符串") "【加标回收】" ("字符串") "【空白校准】" ("字符串") "【标样校准】" ("字符串")] -> w390
                    frame "空闲", Default {
                    }
                    frame "水样测试" {
                    }
                    frame "标样核查" {
                    }
                    frame "零点核查" {
                    }
                    frame "跨度核查" {
                    }
                    frame "空白测试" {
                    }
                    frame "平行样测试" {
                    }
                    frame "加标回收" {
                    }
                    frame "空白校准" {
                    }
                    frame "标样校准" {
                    }
                  }
                  n198 = Format Into String(format string="F0=%#f,F1=%#f,F2=%#f,F3=%#f,Flow=%d-%-d-%-d" ("格式字符串"), w404, w403, w402, w401, w400, w399, w398) -> (resulting string=w405:string)  [unwired: 2 in, 1 out]
                  n199 = Concatenate Strings(w390, w389) -> (w388:string)
                  n200 = Get Date/Time In Seconds() -> (seconds since 1Jan1904=w408:timestamp)
                  n201 = Bundle By Name(cluster=T20 {"时间标识"=timestamp(0 s since 1904-01-01), "设备"="", "日志信息"="", "流程参数"=""} ("data in"), "时间标识"=w408, "设备"=w386, "日志信息"=w388, "流程参数"=w405) -> (w409:T20)
                  n202 = call "总氮操作日志.vi"("data in"=w409) -> ()  [unwired: 11 in]
                }
              }
            }
            n203 = local write "数组"(w366) -> ()
          }
        }
      }
    }
    n204 = case shown="真" w314 {
      tunnel: w294 -> [_ w451]
      frame False {
      }
      frame True {
        n205 = Subtract(x=w451, y=1) -> (x-y=w449:i32)
        n206 = Subtract(x=w449, y=5) -> (x-y=w453:i32)
        n207 = Greater Or Equal To 0?(x=w453) -> (x >= 0?=w452:bool)
        n208 = property on="多列列表框" class="MCListbox (严格)"() -> (error out=w457:errorcluster, "TopLeft"=w458:T21)  [unwired: 2 in, 1 out]
        n209 = Select(t=w453, s=w452, f=0) -> (s? t:f=w454:i32)
        n210 = Bundle By Name(cluster=w458, "Row"=w454) -> (w459:T21)
        n211 = property on="多列列表框" class="MCListbox (严格)"(error in=w457, "TopLeft"=w459) -> ()  [unwired: 1 in, 2 out]
      }
    }
    n212 = call <vilib>:"Boolean Crossing PtByPt.vi"("input"=w312) -> ("crossing"=w287:bool)  [unwired: 2 in]
    n213 = First Call?() -> (First Call?: T/F=w313:bool)
    n214 = case shown="真" w286 {
      tunnel: w284 -> [_ w337]
      tunnel: w280 -> [_ w341]
      frame False {
      }
      frame True {
        n215 = case shown="\"水样测试\"" w341 {
          tunnel: [_ "【水样测试】" ("字符串") "【标样核查】" ("字符串") "【零点核查】" ("字符串") "【跨度核查】" ("字符串") "【空白测试】" ("字符串") "【平行样测试】" ("字符串") "【加标回收】" ("字符串") "【空白校准】" ("字符串") "【标样校准】" ("字符串")] -> w345
          frame "空闲", Default {
          }
          frame "水样测试" {
          }
          frame "标样核查" {
          }
          frame "零点核查" {
          }
          frame "跨度核查" {
          }
          frame "空白测试" {
          }
          frame "平行样测试" {
          }
          frame "加标回收" {
          }
          frame "空白校准" {
          }
          frame "标样校准" {
          }
        }
        n216 = call "id参数转换.vi"("id"=w337) -> ("table输出"=w338:string)  [unwired: 10 in]
        n217 = Concatenate Strings("-->>" ("字符串"), w345, "启动" ("字符串")) -> (w346:string)
        n218 = Get Date/Time In Seconds() -> (seconds since 1Jan1904=w343:timestamp)
        n219 = Bundle By Name(cluster=T20 {"时间标识"=timestamp(0 s since 1904-01-01), "设备"="", "日志信息"="", "流程参数"=""} ("data in"), "时间标识"=w343, "设备"=w338, "日志信息"=w346) -> (w342:T20)
        n220 = call "总氮操作日志.vi"("data in"=w342) -> ()  [unwired: 11 in]
      }
    }
    n221 = case shown="真" w281 {
      tunnel: w284 -> [_ w318]
      tunnel: w280 -> [_ w322]
      frame False {
      }
      frame True {
        n222 = case shown="\"水样测试\"" w322 {
          tunnel: [_ "【水样测试】" ("字符串") "【标样核查】" ("字符串") "【零点核查】" ("字符串") "【跨度核查】" ("字符串") "【空白测试】" ("字符串") "【平行样测试】" ("字符串") "【加标回收】" ("字符串") "【空白校准】" ("字符串") "【标样校准】" ("字符串")] -> w326
          frame "空闲", Default {
          }
          frame "水样测试" {
          }
          frame "标样核查" {
          }
          frame "零点核查" {
          }
          frame "跨度核查" {
          }
          frame "空白测试" {
          }
          frame "平行样测试" {
          }
          frame "加标回收" {
          }
          frame "空白校准" {
          }
          frame "标样校准" {
          }
        }
        n223 = call "id参数转换.vi"("id"=w318) -> ("table输出"=w319:string)  [unwired: 10 in]
        n224 = Concatenate Strings("-->>" ("字符串"), w326, "停止" ("字符串")) -> (w327:string)
        n225 = Get Date/Time In Seconds() -> (seconds since 1Jan1904=w324:timestamp)
        n226 = Bundle By Name(cluster=T20 {"时间标识"=timestamp(0 s since 1904-01-01), "设备"="", "日志信息"="", "流程参数"=""} ("data in"), "时间标识"=w324, "设备"=w319, "日志信息"=w327) -> (w323:T20)
        n227 = call "总氮操作日志.vi"("data in"=w323) -> ()  [unwired: 11 in]
      }
    }
    n228 = Or(x=w287, y=w313) -> (x .or. y?=w311:bool)
    n229 = Bundle By Name(cluster=T19 {"启动模式"=enum."跨度核查", "启动参数"=1, "量程"=enum."低量程"} ("参数簇"), "启动参数"=w307, "启动模式"=w309, "量程"=w308) -> (w301:T19)
    n230 = while {
      tunnel: w311 -> [w437]
      tunnel: w301 -> [w436]
      shift-right: [w431] -> _
      shift-left: _ -> [w433]
      shift-right: [w432] -> _
      shift-left: _ -> [w434]
      shift-right: ["流程路径"] -> _
      shift-left: _ -> [w430]
      stop <- TRUE stop-if-true
      n231 = Not Equal?(x=w430, y="流程路径") -> (x != y?=w427:bool)
      n232 = Or(x=w437, y=w427) -> (x .or. y?=w428:bool)
      n233 = case shown="真" w428 {
        tunnel: [w439 w447] -> w432
        tunnel: [w438 w446] -> w431
        tunnel: w436 -> [_ w441]
        tunnel: w434 -> [w439 _]
        tunnel: w433 -> [w438 _]
        tunnel: "流程路径" -> [_ w440]
        frame False {
        }
        frame True {
          n234 = call "斯坦道XML解析.vi"("添加的路径"=w440, "参数簇"=w441) -> ("步骤时间"=w442:string[], "步骤名"=w444:string[])  [unwired: 8 in]
          n235 = Build Array(w444, w442) -> (w443:string[][])
          n236 = for {
            tunnel: w444 -> [_] mode=indexing
            tunnel: [w448] -> w445 mode=indexing
            i -> [w448]
          }
          n237 = Transpose 2D Array(2D array=w443) -> (transposed array=w446:string[][])
          n238 = Number To Decimal String(number=w445) -> (decimal integer string=w447:string[])  [unwired: 1 in]
        }
      }
      n239 = property on="多列列表框" class="MCListbox (严格)"("ItemNames"=w431, "RowHdrs[]"=w432) -> ()  [unwired: 2 in, 2 out]
    }
    n240 = Wait (ms)(milliseconds to wait=u32 1000 ("等待时间（毫秒）")) -> ()  [unwired: 1 out]
  }
  n241 = Bundle("参数下拉列表"=w12, "测量模式下拉列表"=w11, "量程下拉列表"=w10) -> (w9:T22)  [unwired: 1 in]
  n242 = property on="曲线模型" class="曲线模型 (严格)"("属性"=w9) -> (error out=w17:errorcluster)  [unwired: 2 in, 1 out]
  n243 = control-ref of="量程参数读取"() -> (w13:refnum<vi>)
  n244 = control-ref of="公式"() -> (w22:refnum<vi>)
  n245 = control-ref of="参数下拉列表"() -> (w24:refnum<vi>)
  n246 = control-ref of="测量模式下拉列表"() -> (w23:refnum<vi>)
  n247 = control-ref of="量程下拉列表"() -> (w25:refnum<vi>)
  n248 = Obtain Notifier(name (unnamed)="TN" ("名称（未命名）"), notification data type=FALSE) -> (notifier out=w14:refnum<notifier>)  [unwired: 2 in, 2 out]
  n249 = Obtain Queue(name (unnamed)="TN" ("名称（未命名）"), element data type=cluster{"命令":string, "data":variant} {"命令"="", "data"=variant}) -> (queue out=w26:refnum<queue>, error out=w27:errorcluster)  [unwired: 3 in, 1 out]
  n250 = while {
    tunnel: w26 -> [w467]
    tunnel: w27 -> [_]
    stop <- FALSE stop-if-true
    n251 = Get Queue Status(queue=w467) -> (queue out=w463:refnum<queue>, # elements in queue=w462:i32)  [unwired: 2 in, 6 out]
    n252 = global read "总氮断电保存全局变量.vi" "流程路径"() -> (w466:path)
    n253 = global read "总氮断电保存全局变量.vi" "MB通信方式选择"() -> (w464:enum16{"串口", "TCP"})
    n254 = case shown="0" w462 {
      tunnel: w463 -> [_ w473]
      frame Default {
      }
      frame 0 {
        w482 = u16 2 items=["总磷"=1, "总氮"=2, "氨氮"=3] ("站号")
        # "试剂填充 172 \n管路清洗108\n氨氮92\n总磷131\n总磷海水147\n总氮76\n总氮海水92"
        n255 = global read "VAR总氮全局变量.vi" "状态告警区"() -> (w474:T9)
        n256 = Unbundle By Name(w474) -> ("系统时间"=w481:timestamp, "工作状态"=w472:T10)
        n257 = Bundle By Name(cluster=cluster{"命令":string, "data":variant} {"命令"="", "data"=variant} ("元素"), "命令"="读状态告警区", "data"=w482) -> (w485:cluster{"命令":string, "data":variant})
        n258 = Get Date/Time In Seconds() -> (seconds since 1Jan1904=w480:timestamp)
        n259 = Enqueue Element(queue=w473, element=w485) -> (queue out=w483:refnum<queue>)  [unwired: 2 in, 2 out]
        n260 = Subtract(x=w480, y=w481) -> (x-y=w479:dbl)
        n261 = Equal?(x=w472, y=T10."空闲") -> (x = y?=w470:bool)
        n262 = Absolute Value(x=w479) -> (abs(x)=w478:dbl)
        n263 = case shown="真" w470 {
          tunnel: w483 -> [w487 w490]
          tunnel: w482 -> [_ w489]
          tunnel: [w487 w488] -> w475
          frame False {
          }
          frame True {
            n264 = Bundle By Name(cluster=cluster{"命令":string, "data":variant} {"命令"="", "data"=variant} ("元素"), "命令"="读测量数据区", "data"=w489) -> (w492:cluster{"命令":string, "data":variant})
            n265 = Enqueue Element(queue=w490, element=w492) -> (queue out=w488:refnum<queue>)  [unwired: 2 in, 2 out]
          }
        }
        n266 = Greater Or Equal?(x=w478, y=120.0) -> (x >= y?=w476:bool)
        n267 = case shown="真" w476 {
          tunnel: w475 -> [_ w495]
          frame False {
          }
          frame True {
            n268 = call "总氮启动命令.vi"("参数"=T23 {"站号"=3, "量程切换"=enum."AUTO", "控制命令"=enum."校时", "模式设置"=enum."待机", "测量间隔"=0}) -> ("启动命令"=w494:cluster{"命令":string, "data":variant})  [unwired: 10 in]
            n269 = Enqueue Element(queue=w495, element=w494) -> ()  [unwired: 2 in, 3 out]
          }
        }
      }
    }
    n270 = local write "流程路径"(w466) -> ()
    n271 = case shown="\"TCP\"" w464 {
      tunnel: [w497 w498] -> w465
      frame "串口", Default {
        n272 = global read "总氮断电保存全局变量.vi" "VISA Resource"() -> (w497:refnum<visa-resource-name>)
      }
      frame "TCP" {
        n273 = global read "总氮断电保存全局变量.vi" "IP"() -> (w498:string)
      }
    }
    "字符串" <- w465
    n274 = Wait (ms)(milliseconds to wait=u32 1000 ("等待时间（毫秒）")) -> ()  [unwired: 1 out]
    n275 = global read "总氮断电保存全局变量.vi" "远程校准量程"() -> (w460:enum16{"低量程", "高量程"})
    n276 = global read "总氮断电保存全局变量.vi" "远程标样校准"() -> (w461:enum16{"标液1", "标液2", "标液3", "标液4"})
    n277 = local write "远程标样校准"(w461) -> ()
    n278 = local write "远程校准量程"(w460) -> ()
  }
  n279 = while {
    tunnel: w26 -> [w505]
    tunnel: w25 -> [w504]
    tunnel: w24 -> [w503]
    tunnel: w23 -> [w502]
    tunnel: w22 -> [w501]
    tunnel: w13 -> [w500]
    tunnel: w17 -> [_]
    tunnel: w14 -> [w499]
    stop <- FALSE stop-if-true
    n280 = event shown="[16] \"设置\": 值改变" {
      selector: _ -> [_ _ _ _ _ _ _ _ _ _ _ _ _ _ _ _ _ _ _ _ _ _ _]
      dyn-events: _ -> [_ _ _ _ _ _ _ _ _ _ _ _ _ _ _ _ _ _ _ _ _ _ _]
      timeout: _ -> [_ _ _ _ _ _ _ _ _ _ _ _ _ _ _ _ _ _ _ _ _ _ _]
      tunnel: w505 -> [_ _ _ _ w533 _ w549 _ _ _ _ _ w610 _ w629 w664 _ _ _ _ _ _ _]
      tunnel: w504 -> [_ _ _ w511 _ _ _ _ _ _ _ _ _ _ _ _ w670 _ _ w693 w696 _ _]
      tunnel: w503 -> [_ _ _ w513 _ _ _ _ _ _ _ _ _ _ _ _ w672 _ _ w691 w698 w754 w761]
      tunnel: w502 -> [_ _ _ w512 _ _ _ _ _ _ _ _ _ _ _ _ w671 _ _ w692 w697 _ _]
      tunnel: w501 -> [_ _ _ w514 _ _ _ _ _ _ _ _ _ _ _ _ w673 _ _ w687 _ _ _]
      tunnel: w500 -> [_ _ _ _ _ _ _ _ _ _ _ _ _ _ _ _ w667 _ _ _ _ w752 _]
      tunnel: w499 -> [_ _ _ _ _ _ _ _ _ _ _ _ _ _ _ w660 _ _ _ _ _ _ _]
      tunnel: [_ _ _ w519 _ _ _ _ _ _ _ _ _ _ _ _ _ _ _ _ _ _ _] -> _
      event Timeout {
        n281 = event-data() -> ()  [unwired: 1 in, 3 out]
      }
      event "流程固件": Value Change {
        # "试剂填充 172 \n管路清洗108\n氨氮92\n总磷131\n总磷海水147\n总氮76\n总氮海水92"
        n282 = event-data() -> ()  [unwired: 1 in, 6 out]
        n283 = call "流程固件设置对话框.vi"() -> ()  [unwired: 12 in]
      }
      event "布尔": Mouse Down {
        n284 = event-data() -> ("CtlRef"=w508:refnum<vi>)  [unwired: 1 in, 5 out]
        n285 = property class="Bool (严格)"(reference=w508) -> ("Value"=w507:bool)  [unwired: 1 in, 2 out]
        n286 = case shown="假" w507 {
          frame False {
            n287 = call "密码键盘.vi"() -> ("NewNumber"=→"输入密码":dbl)  [unwired: 1 in]
          }
          frame True {
            n288 = local write "输入密码"(u32 0 ("输入密码")) -> ()
          }
        }
      }
      event "测量模式下拉列表", "量程下拉列表", "参数下拉列表": Value Change {
        n289 = event-data() -> ()  [unwired: 1 in, 6 out]
        n290 = property class="Enum (严格)"(reference=w513) -> ("Value"=w518:enum16{"总磷", "总氮"})  [unwired: 1 in, 2 out]
        n291 = property class="Enum (严格)"(reference=w512) -> ("Value"=w517:enum16{"水样测量", "零点核查", "跨度核查", "标样核查", "加标回收"})  [unwired: 1 in, 2 out]
        n292 = property class="Enum (严格)"(reference=w511) -> ("Value"=w516:enum16{"低量程", "高量程"})  [unwired: 1 in, 2 out]
        n293 = call "总磷总氮公式读取.vi"("量程"=w516, "测量模式"=w517, "测量参数"=w518) -> ("公式"=w515:cluster{"X^2":dbl, "X":dbl, "b":dbl})  [unwired: 7 in, 1 out]
        n294 = property class="Clust (严格)"(reference=w514, "Value"=w515) -> ()  [unwired: 1 in, 2 out]
        n295 = local read "参数下拉列表"() -> (w520:enum16{"总磷", "总氮"})
        n296 = local read "测量模式下拉列表"() -> (w521:enum16{"水样测量", "零点核查", "跨度核查", "标样核查", "加标回收"})
        n297 = local read "量程下拉列表"() -> (w522:enum16{"低量程", "高量程"})
        n298 = Bundle("参数下拉列表"=w520, "测量模式下拉列表"=w521, "量程下拉列表"=w522) -> (w523:T22)  [unwired: 1 in]
        n299 = property on="曲线模型" class="曲线模型 (严格)"("属性"=w523) -> (error out=w519:errorcluster)  [unwired: 2 in, 1 out]
      }
      event "串口设置": Value Change {
        n300 = event-data() -> ()  [unwired: 1 in, 6 out]
        n301 = global read "总氮断电保存全局变量.vi" "VISA Resource"() -> (w530:refnum<visa-resource-name>)
        n302 = global read "总氮断电保存全局变量.vi" "MB通信方式选择"() -> (w524:enum16{"串口", "TCP"})
        n303 = global read "总氮断电保存全局变量.vi" "IP"() -> (w525:string)
        n304 = global read "总氮断电保存全局变量.vi" "PORT"() -> (w529:string)
        n305 = call "串口配置.vi"("PORT"=w529, "IP"=w525, "MB通信方式选择"=w524, "请选择串口:"=w530) -> ("PORT 2"=w527:string, "IP 2"=w528:string, "确认 2"=w531:bool, "VISA资源名称 2"=w532:refnum<visa-resource-name>, "MB通信方式选择 2"=w526:enum16{"串口", "TCP"})  [unwired: 3 in]
        n306 = case shown="真" w531 {
          tunnel: w532 -> [_ w538]
          tunnel: w533 -> [_ w537]
          tunnel: w528 -> [_ w536]
          tunnel: w527 -> [_ w535]
          tunnel: w526 -> [_ w534]
          frame False {
          }
          frame True {
            n307 = flat-sequence {
              tunnel: w538 -> [w543]
              tunnel: w537 -> [w544]
              tunnel: w536 -> [w542]
              tunnel: w535 -> [w541]
              tunnel: w534 -> [w540]
              frame #0 {
                n308 = global write "总氮断电保存全局变量.vi" "IP"(w542) -> ()
                n309 = global write "总氮断电保存全局变量.vi" "PORT"(w541) -> ()
                n310 = global write "总氮断电保存全局变量.vi" "MB通信方式选择"(w540) -> ()
                n311 = global write "总氮断电保存全局变量.vi" "VISA Resource"(w543) -> ()
                n312 = Flush Queue(queue=w544) -> (queue out=w539:refnum<queue>)  [unwired: 1 in, 2 out]
                n313 = Enqueue Element(queue=w539, element=cluster{"命令":string, "data":variant} {"命令"="启用模块", "data"=variant} ("元素")) -> ()  [unwired: 2 in, 3 out]
              }
              frame #1 {
                n314 = call "配置文件保存.vi"() -> ()  [unwired: 12 in]
              }
            }
          }
        }
      }
      event "远程校准量程", "远程标样校准": Value Change {
        n315 = event-data() -> ()  [unwired: 1 in, 6 out]
        n316 = flat-sequence {
          frame #0 {
            n317 = global write "总氮断电保存全局变量.vi" "远程标样校准"("远程标样校准") -> ()
            n318 = global write "总氮断电保存全局变量.vi" "远程校准量程"("远程校准量程") -> ()
          }
          frame #1 {
            n319 = call "配置文件保存.vi"() -> ()  [unwired: 12 in]
          }
        }
      }
      event "模块启用": Value Change {
        n320 = event-data() -> ("OldVal"=w550:bool)  [unwired: 1 in, 5 out]
        n321 = Flush Queue(queue=w549) -> (queue out=w548:refnum<queue>)  [unwired: 1 in, 2 out]
        n322 = case shown="假" w550 {
          tunnel: w548 -> [w551 w553]
          frame False {
            n323 = Enqueue Element(queue=w551, element=cluster{"命令":string, "data":variant} {"命令"="停用模块", "data"=variant} ("元素")) -> ()  [unwired: 2 in, 3 out]
          }
          frame True {
            n324 = Enqueue Element(queue=w553, element=cluster{"命令":string, "data":variant} {"命令"="启用模块", "data"=variant} ("元素")) -> ()  [unwired: 2 in, 3 out]
          }
        }
      }
      event "流程路径": Value Change {
        n325 = event-data() -> ()  [unwired: 1 in, 6 out]
        n326 = flat-sequence {
          frame #0 {
            n327 = local read "流程路径"() -> (w555:path)
            n328 = global write "总氮断电保存全局变量.vi" "流程路径"(w555) -> ()
          }
          frame #1 {
            n329 = call "配置文件保存.vi"() -> ()  [unwired: 12 in]
          }
        }
      }
      event "公式一键写入": Value Change {
        n330 = event-data() -> ()  [unwired: 1 in, 6 out]
        n331 = local read "公式"() -> (w556:cluster{"X^2":dbl, "X":dbl, "b":dbl})
        n332 = call "公式复合写入.vi"("公式"=w556) -> ()  [unwired: 11 in]
      }
      event "曲线模型": Value Change {
        n333 = event-data() -> ()  [unwired: 1 in, 6 out]
        n334 = disable-structure shown="禁用" {
          frame Disabled {
            n335 = Unbundle By Name("曲线模型") -> ("X^2"=w559:dbl, "X"=w560:dbl, "B"=w561:dbl)
            n336 = Build Array(w559, w560, w561) -> (w558:dbl[])
            n337 = Array To Cluster(array=w558) -> (cluster=w557:cluster{"[0]":dbl, "[1]":dbl, "[2]":dbl})
            n338 = local write "公式"(w557) -> ()
          }
          frame Enabled {
          }
        }
      }
      event "质控参数设置": Value Change {
        n339 = event-data() -> ()  [unwired: 1 in, 6 out]
        n340 = global read "总氮断电保存全局变量.vi" "总氮自动测试量程配置"() -> (w564:T24)
        n341 = global read "总氮断电保存全局变量.vi" "质控参数设置"() -> (w565:T25)
        n342 = call "总氮质控参数设置.vi"("自动测试量程配置"=w564, "质控参数设置"=w565) -> ("自动测试量程配置输出"=w563:T24, "输出簇"=w566:T26)  [unwired: 8 in]
        n343 = Unbundle By Name(w566) -> ("确定"=w567:bool)
        n344 = case shown="真" w567 {
          tunnel: w566 -> [_ w570]
          tunnel: w565 -> [_ w569]
          tunnel: w563 -> [_ w568]
          frame False {
          }
          frame True {
            n345 = flat-sequence {
              tunnel: w570 -> [w578]
              tunnel: w569 -> [w577]
              tunnel: w568 -> [w571]
              frame #0 {
                n346 = Unbundle By Name(w578) -> ("跨度值"=w576:dbl, "零点标准液浓度"=w575:dbl, "跨度标准液浓度"=w574:dbl, "标准液标准浓度"=w573:dbl)
                n347 = global write "总氮断电保存全局变量.vi" "总氮自动测试量程配置"(w571) -> ()
                n348 = Bundle By Name(cluster=w577, "跨度值"=w576, "零点标准液浓度"=w575, "跨度标准液浓度"=w574, "标准液标准浓度"=w573) -> (w572:T25)
                n349 = global write "总氮断电保存全局变量.vi" "质控参数设置"(w572) -> ()
              }
              frame #1 {
                n350 = call "配置文件保存.vi"() -> ()  [unwired: 12 in]
              }
            }
          }
        }
      }
      event "仪器参数设置": Value Change {
        n351 = event-data() -> ()  [unwired: 1 in, 6 out]
        n352 = global read "总氮断电保存全局变量.vi" "总氮仪器参数"() -> (w579:T27)
        n353 = call "仪器参数设置.vi"("氨氮仪器参数"=w579) -> ("仪器参数设置输出"=w580:T28)  [unwired: 10 in]
        n354 = Unbundle By Name(w580) -> ("确定"=w581:bool)
        n355 = case shown="真" w581 {
          tunnel: w580 -> [_ w583]
          tunnel: w579 -> [_ w582]
          frame False {
          }
          frame True {
            n356 = flat-sequence {
              tunnel: w583 -> [w600]
              tunnel: w582 -> [w599]
              frame #0 {
                n357 = Unbundle By Name(w600) -> ("测量量程"=w598:dbl, "测量精度"=w597:dbl, "测量间隔"=w596:dbl, "消解温度"=w595:dbl, "消解时长"=w593:dbl, "空白校准时间"=w592:timestamp, "曲线截距"=w591:dbl, "曲线斜率"=w590:dbl, "测量检出限"=w589:dbl, "测量信号值"=w588:dbl, "线性相关系数"=w587:dbl, "二次多项式系数"=w586:dbl, "标样校准时间"=w585:timestamp, "稀释倍数"=w584:dbl)
                n358 = Bundle By Name(cluster=w599, "测量量程"=w598, "测量精度"=w597, "测量间隔"=w596, "消解温度"=w595, "消解时长"=w593, "空白校准时间"=w592, "曲线截距"=w591, "曲线斜率"=w590, "测量检出限"=w589, "测量信号值"=w588, "线性相关系数"=w587, "二次多项式系数"=w586, "标样校准时间"=w585, "稀释倍数"=w584) -> (w594:T27)
                n359 = global write "总氮断电保存全局变量.vi" "总氮仪器参数"(w594) -> ()
              }
              frame #1 {
                n360 = call "配置文件保存.vi"() -> ()  [unwired: 12 in]
              }
            }
          }
        }
      }
      event "手动启动": Value Change {
        n361 = event-data() -> ()  [unwired: 1 in, 6 out]
        n362 = call "总氮启动参数对话框.vi"() -> ("标样浓度输出"=w602:dbl, "确认"=w609:bool, "元素"=w603:cluster{"命令":string, "data":variant})  [unwired: 9 in]
        n363 = case shown="真" w609 {
          tunnel: w610 -> [_ w625]
          tunnel: w603 -> [_ w624]
          frame False {
          }
          frame True {
            n364 = Enqueue Element(queue=w625, element=w624) -> ()  [unwired: 2 in, 3 out]
          }
        }
        n365 = Unbundle By Name(w603) -> ("data"=w607:variant)
        n366 = Variant To Data(type=cluster{"站号":u16, "控制命令":u16[]} {"站号"=0, "控制命令"=[]} ("输出簇"), Variant=w607) -> (data=w606:cluster{"站号":u16, "控制命令":u16[]})  [unwired: 1 in, 1 out]
        n367 = Unbundle By Name(w606) -> ("控制命令"=w605:u16[])
        n368 = Index Array(array=w605) -> (element=w604:u16)  [unwired: 1 in]
        n369 = Swap Bytes(anything=w604) -> (byte swapped=w601:u16)
        n370 = case shown="0, 默认" w601 {
          tunnel: w602 -> [_ w618 _]
          frame 0, Default {
            n371 = local read "远程标样校准"() -> (w613:enum16{"标液1", "标液2", "标液3", "标液4"})
            n372 = case shown="\"标液4\"" w613 {
              tunnel: TRUE ("值(信号)") -> [w614 w615 w616 w617]
              frame "标液1", Default {
                n373 = property on="校准2" class="Bool (严格)"("Val(Sgnl)"=w614) -> ()  [unwired: 2 in, 2 out]
              }
              frame "标液2" {
                n374 = property on="校准3" class="Bool (严格)"("Val(Sgnl)"=w615) -> ()  [unwired: 2 in, 2 out]
              }
              frame "标液3" {
                n375 = property on="校准4" class="Bool (严格)"("Val(Sgnl)"=w616) -> ()  [unwired: 2 in, 2 out]
              }
              frame "标液4" {
                n376 = property on="校准5" class="Bool (严格)"("Val(Sgnl)"=w617) -> ()  [unwired: 2 in, 2 out]
              }
            }
            n377 = local read "远程校准量程"() -> (w611:enum16{"低量程", "高量程"})
            n378 = property on="量程下拉列表" class="Enum (严格)"("Val(Sgnl)"=w611) -> ()  [unwired: 2 in, 2 out]
          }
          frame 2 {
            n379 = flat-sequence {
              tunnel: w618 -> [w620]
              frame #0 {
                n380 = global read "总氮断电保存全局变量.vi" "质控参数设置"() -> (w621:T25)
                n381 = Bundle By Name(cluster=w621, "标准液标准浓度"=w620) -> (w619:T25)
                n382 = global write "总氮断电保存全局变量.vi" "质控参数设置"(w619) -> ()
              }
              frame #1 {
                n383 = call "配置文件保存.vi"() -> ()  [unwired: 12 in]
              }
            }
          }
          frame 8 {
            # "空白校准"
            n384 = property on="校准1" class="Bool (严格)"("Val(Sgnl)"=TRUE ("值(信号)")) -> ()  [unwired: 2 in, 2 out]
            n385 = property on="量程下拉列表" class="Enum (严格)"("Val(Sgnl)"=enum16{"低量程", "高量程"}."低量程" ("值(信号)")) -> ()  [unwired: 2 in, 2 out]
          }
        }
      }
      event "单步测试": Value Change {
        n386 = event-data() -> ()  [unwired: 1 in, 6 out]
        n387 = call "总氮单步调试对话框.vi"() -> ()  [unwired: 12 in]
      }
      event "校准按钮.校准1", "校准按钮.校准2", "校准按钮.校准3", "校准按钮.校准4", "校准按钮.校准5": Value Change {
        n388 = event-data() -> ("CtlRef"=w635:refnum<vi>)  [unwired: 1 in, 5 out]
        n389 = property class="Bool (严格)"(reference=w635) -> ("Label.Text"=w633:string)  [unwired: 1 in, 2 out]
        n390 = property on="曲线模型" class="曲线模型 (严格)"() -> ("浓度属性"=w634:T29)  [unwired: 2 in, 2 out]
        n391 = case shown="\"校准3\"" w633 {
          tunnel: [w643 w646 w649 w652 w655] -> w631
          tunnel: [u16 1 ("校准点1-5") u16 2 ("校准点1-5") u16 3 ("校准点1-5") u16 4 ("校准点1-5") u16 5 ("校准点1-5")] -> w632
          tunnel: w634 -> [w644 w647 w650 w653 w656]
          frame "校准1", Default {
            n392 = Unbundle By Name(w644) -> ("标液浓度1"=w643:dbl)
          }
          frame "校准2" {
            n393 = Unbundle By Name(w647) -> ("标液浓度2"=w646:dbl)
          }
          frame "校准3" {
            n394 = Unbundle By Name(w650) -> ("标液浓度3"=w649:dbl)
          }
          frame "校准4" {
            n395 = Unbundle By Name(w653) -> ("标液浓度4"=w652:dbl)
          }
          frame "校准5" {
            n396 = Unbundle By Name(w656) -> ("标液浓度5"=w655:dbl)
          }
        }
        n397 = Not Equal To 0?(x=w631) -> (x != 0?=w627:bool)
        n398 = Bundle By Name(cluster=cluster{"校准？":bool, "校准点1-5":u16, "校准浓度":dbl} {"校准？"=FALSE, "校准点1-5"=0, "校准浓度"=0.0} ("校准输出"), "校准？"=TRUE, "校准点1-5"=w632, "校准浓度"=w631) -> (w630:cluster{"校准？":bool, "校准点1-5":u16, "校准浓度":dbl})
        n399 = global write "总氮断电保存全局变量.vi" "校准输出"(w630) -> ()
        n400 = local read "量程下拉列表"() -> (w626:enum16{"低量程", "高量程"})
        n401 = case shown="真" w627 {
          tunnel: [cluster{"命令":string, "data":variant} {"命令"="启动", "data"=variant(cluster{"站号":u16, "控制命令":u16[]} {"站号"=2, "控制命令"=[2048, 256]})} ("元素") w639] -> w628
          tunnel: w626 -> [_ w640]
          frame False {
            # "校零"
          }
          frame True {
            # "校标"
            n402 = case shown="\"低量程\", 默认" w640 {
              tunnel: [cluster{"命令":string, "data":variant} {"命令"="启动", "data"=variant(cluster{"站号":u16, "控制命令":u16[]} {"站号"=2, "控制命令"=[2304, 256]})} ("元素") cluster{"命令":string, "data":variant} {"命令"="启动", "data"=variant(cluster{"站号":u16, "控制命令":u16[]} {"站号"=2, "控制命令"=[2304, 257]})} ("元素")] -> w639
              frame "低量程", Default {
              }
              frame "高量程" {
              }
            }
          }
        }
        n403 = Enqueue Element(queue=w629, element=w628) -> ()  [unwired: 2 in, 3 out]
      }
      event "停止": Value Change {
        n404 = event-data() -> ()  [unwired: 1 in, 6 out]
        n405 = Cancel Notification(0:w660) -> (8:w659:refnum<notifier>)  [unwired: 1 in, 2 out]
        n406 = Enqueue Element(queue=w664, element=cluster{"命令":string, "data":variant} {"命令"="启动", "data"=variant(cluster{"站号":u16, "控制命令输出":u16[]} {"站号"=1, "控制命令输出"=[2816]})} ("元素")) -> (queue out=w661:refnum<queue>)  [unwired: 2 in, 2 out]
        n407 = Send Notification(notification=TRUE ("通知"), notifier=w659) -> ()  [unwired: 1 in, 2 out]
        n408 = Enqueue Element(queue=w661, element=cluster{"命令":string, "data":variant} {"命令"="启动", "data"=variant(cluster{"站号":u16, "控制命令输出":u16[]} {"站号"=2, "控制命令输出"=[2816]})} ("元素")) -> ()  [unwired: 2 in, 3 out]
      }
      event "设置": Value Change {
        n409 = event-data() -> ()  [unwired: 1 in, 6 out]
        n410 = property class="Enum (严格)"(reference=w672) -> (reference out=w666:refnum<vi>, "Value"=w677:enum16{"总磷", "总氮"})  [unwired: 1 in, 1 out]
        n411 = property class="Enum (严格)"(reference=w671) -> ("Value"=w676:enum16{"水样测量", "零点核查", "跨度核查", "标样核查", "加标回收"})  [unwired: 1 in, 2 out]
        n412 = property class="Enum (严格)"(reference=w670) -> ("Value"=w675:enum16{"低量程", "高量程"})  [unwired: 1 in, 2 out]
        n413 = property on="窗格" class="Pane"("Origin"=T7 {"Horizontal"=0, "Vertical"=628} ("原点")) -> ()  [unwired: 2 in, 2 out]
        n414 = call "总磷总氮公式读取.vi"("量程"=w675, "测量模式"=w676, "测量参数"=w677) -> ("error out"=w665:errorcluster, "公式"=w674:cluster{"X^2":dbl, "X":dbl, "b":dbl})  [unwired: 7 in]
        n415 = property class="Clust (严格)"(reference=w673, "Value"=w674) -> ()  [unwired: 1 in, 2 out]
        n416 = property class="Enum (严格)"(reference=w666) -> ("Value"=w669:enum16{"总磷", "总氮"})  [unwired: 1 in, 2 out]
        n417 = call "总磷总氮量程读取.vi"("error in (no error)"=w665, "测量参数"=w669) -> ("量程参数读取"=w668:T30)  [unwired: 8 in, 1 out]
        n418 = property class="Clust (严格)"(reference=w667, "Value"=w668) -> ()  [unwired: 1 in, 2 out]
      }
      event "返回": Value Change {
        n419 = event-data() -> ()  [unwired: 1 in, 6 out]
        n420 = property on="窗格" class="Pane"("Origin"=T7 {"Horizontal"=0, "Vertical"=0} ("原点")) -> ()  [unwired: 2 in, 2 out]
      }
      event "公式.X^2", "公式.X", "公式.b", "量程参数读取.测量精度", "量程参数读取.检出限", "量程参数读取.上限", "量程参数读取.下限", "量程参数读取.(低->高)", "量程参数读取.(高->低)", "量程参数读取.稀释度": Mouse Down {
        n421 = event-data() -> ("CtlRef"=w683:refnum<vi>)  [unwired: 1 in, 5 out]
        n422 = property class="DigNum (严格)"(reference=w683) -> (reference out=w681:refnum<vi>, "Value"=w682:dbl)  [unwired: 1 in, 1 out]
        n423 = call "数字键盘.vi"("OldNumber"=w682) -> ("NewNumber"=w680:dbl)
        n424 = property class="DigNum (严格)"(reference=w681, "Val(Sgnl)"=w680) -> ()  [unwired: 1 in, 2 out]
      }
      event "读公式": Value Change {
        n425 = event-data() -> ()  [unwired: 1 in, 6 out]
        n426 = property class="Enum (严格)"(reference=w691) -> ("Value"=w690:enum16{"总磷", "总氮"})  [unwired: 1 in, 2 out]
        n427 = property class="Enum (严格)"(reference=w692) -> ("Value"=w689:enum16{"水样测量", "零点核查", "跨度核查", "标样核查", "加标回收"})  [unwired: 1 in, 2 out]
        n428 = property class="Enum (严格)"(reference=w693) -> ("Value"=w688:enum16{"低量程", "高量程"})  [unwired: 1 in, 2 out]
        n429 = call "总磷总氮公式读取.vi"("量程"=w688, "测量模式"=w689, "测量参数"=w690) -> ("error out"=w685:errorcluster, "公式"=w686:cluster{"X^2":dbl, "X":dbl, "b":dbl})  [unwired: 7 in]
        n430 = property class="Clust (严格)"(reference=w687, "Value"=w686) -> ()  [unwired: 1 in, 2 out]
        n431 = case shown="错误" w685 {
          tunnel: ["读取成功" ("消息") "读取失败" ("消息")] -> w684
          frame No Error {
          }
          frame Error {
          }
        }
        n432 = One Button Dialog(message=w684) -> ()  [unwired: 1 in, 1 out]
      }
      event "写公式": Value Change {
        n433 = event-data() -> ()  [unwired: 1 in, 6 out]
        n434 = call <vilib>:"Three Button Dialog.vi"("Allow user to close window? (TRUE)"=FALSE, "Center Button Text (\"No\")"="一键写入所有公式" ("F按钮名称（“取消”）"), "Left Button Text (\"Yes\")"="写入当前公式" ("T按钮名称（“确定”）"), "message"="即将将左侧拟合公式写入仪器\n请选择写入当前模式还是一键写入所有模式！" ("消息")) -> ("Which Button?"=w699:T31)  [unwired: 7 in]
        n435 = case shown="\"Center Button\"" w699 {
          tunnel: w698 -> [w709 w742 _ _]
          tunnel: w697 -> [w708 w741 _ _]
          tunnel: w696 -> [w707 w740 _ _]
          frame "Left Button", Default {
            n436 = local read "曲线模型"() -> (w715:cluster{"X^2":dbl, "X":dbl, "B":dbl, "r^2":dbl})
            n437 = Unbundle By Name(w715) -> ("X^2"=w713:dbl, "X"=w712:dbl, "B"=w711:dbl)
            n438 = Build Array(w713, w712, w711) -> (w714:dbl[])
            n439 = Array To Cluster(array=w714) -> (cluster=w710:cluster{"[0]":dbl, "[1]":dbl, "[2]":dbl})
            n440 = call "总磷总氮公式写入.vi"("公式"=w710, "量程"="量程下拉列表", "测量模式"="测量模式下拉列表", "测量参数"="参数下拉列表") -> ("error out"=w719:errorcluster)  [unwired: 7 in]
            n441 = call "公式发生改变存储 (子VI).vi"("公式"=w710, "量程下拉列表输入"=w707, "测量模式下拉列表输入"=w708, "参数"=w709) -> ()  [unwired: 8 in]
            n442 = local write "公式"(w710) -> ()
            n443 = case shown="无错误" w719 {
              tunnel: ["写入成功" ("消息") "写入失败" ("消息")] -> w720
              tunnel: "测量模式下拉列表" -> [w723 _]
              tunnel: "量程下拉列表" -> [w722 _]
              tunnel: w710 -> [w721 _]
              frame No Error {
                n444 = Equal?(x=w723, y=enum16{"水样测量", "零点核查", "跨度核查", "标样核查", "加标回收"}."水样测量") -> (x = y?=w726:bool)
                n445 = Equal?(x=w722, y=enum16{"低量程", "高量程"}."低量程") -> (x = y?=w725:bool)
                n446 = Compound Arithmetic op=AND ("复合运算")(w726, w725) -> (w724:bool)
                n447 = case shown="真" w724 {
                  tunnel: w721 -> [_ w735]
                  frame False {
                  }
                  frame True {
                    n448 = Unbundle By Name(w735) -> ("[0]"=w732:dbl, "[1]"=w734:dbl, "[2]"=w733:dbl)
                    n449 = global read "总氮断电保存全局变量.vi" "总氮仪器参数"() -> (w731:T27)
                    n450 = Bundle By Name(cluster=w731, "曲线截距"=w733, "曲线斜率"=w734, "二次多项式系数"=w732) -> (w730:T27)
                    n451 = global write "总氮断电保存全局变量.vi" "总氮仪器参数"(w730) -> ()
                  }
                }
              }
              frame Error {
              }
            }
            n452 = control-ref of="曲线模型"() -> (w705:refnum<vi>)
            n453 = control-ref of="量程下拉列表"() -> (w704:refnum<vi>)
            n454 = call "生成校准信息.vi"("table输入"="总氮", "量程下拉列表"=w704, "曲线模型"=w705) -> ()  [unwired: 9 in]
            n455 = One Button Dialog(message=w720) -> ()  [unwired: 1 in, 1 out]
          }
          frame "Center Button" {
            n456 = local read "曲线模型"() -> (w748:cluster{"X^2":dbl, "X":dbl, "B":dbl, "r^2":dbl})
            n457 = Unbundle By Name(w748) -> ("X^2"=w746:dbl, "X"=w745:dbl, "B"=w744:dbl)
            n458 = Build Array(w746, w745, w744) -> (w747:dbl[])
            n459 = Array To Cluster(array=w747) -> (cluster=w743:cluster{"[0]":dbl, "[1]":dbl, "[2]":dbl})
            n460 = local write "公式"(w743) -> ()
            n461 = call "公式复合写入.vi"("公式"=w743) -> ()  [unwired: 11 in]
            n462 = call "公式发生改变存储 (子VI).vi"("公式"=w743, "量程下拉列表输入"=w740, "测量模式下拉列表输入"=w741, "参数"=w742) -> ()  [unwired: 8 in]
            n463 = control-ref of="曲线模型"() -> (w738:refnum<vi>)
            n464 = control-ref of="量程下拉列表"() -> (w737:refnum<vi>)
            n465 = call "生成校准信息.vi"("table输入"="总氮", "量程下拉列表"=w737, "曲线模型"=w738) -> ()  [unwired: 9 in]
          }
          frame "Right Button" {
          }
          frame "Window Close" {
          }
        }
      }
      event "量程切换阈值读取": Value Change {
        n466 = event-data() -> ()  [unwired: 1 in, 6 out]
        n467 = property class="Enum (严格)"(reference=w754) -> ("Value"=w753:enum16{"总磷", "总氮"})  [unwired: 1 in, 2 out]
        n468 = call "总磷总氮量程读取.vi"("测量参数"=w753) -> ("error out"=w749:errorcluster, "量程参数读取"=w751:T30)  [unwired: 9 in]
        n469 = property class="Clust (严格)"(reference=w752, "Value"=w751) -> ()  [unwired: 1 in, 2 out]
        n470 = case shown="错误" w749 {
          tunnel: ["读取成功" ("消息") "读取失败" ("消息")] -> w750
          frame No Error {
          }
          frame Error {
          }
        }
        n471 = One Button Dialog(message=w750) -> ()  [unwired: 1 in, 1 out]
      }
      event "量程切换阈值写入": Value Change {
        n472 = event-data() -> ()  [unwired: 1 in, 6 out]
        n473 = property class="Enum (严格)"(reference=w761) -> ("Value"=w760:enum16{"总磷", "总氮"})  [unwired: 1 in, 2 out]
        n474 = call "总磷总氮量程写入.vi"("量程参数写入"="量程参数读取", "测量参数"=w760) -> ("error out"=w758:errorcluster)  [unwired: 8 in]
        n475 = case shown="无错误" w758 {
          tunnel: ["写入成功" ("消息") "写入失败" ("消息")] -> w759
          frame No Error {
          }
          frame Error {
          }
        }
        n476 = One Button Dialog(message=w759) -> ()  [unwired: 1 in, 1 out]
      }
    }
  }
  n477 = while {
    tunnel: [w771] -> _
    shift-right: [w769] -> _
    shift-left: w7 -> [w768]
    tunnel: w4 -> [w765]
    stop <- FALSE stop-if-true
    n478 = global read "VAR总氮全局变量.vi" "配置文件 path"() -> (w764:path)
    n479 = Read from Text File(file (use dialog)=w764, error in=w765) -> (text=w769:string, error out=w766:errorcluster)  [unwired: 2 in, 2 out]
    n480 = Not Equal?(x=w769, y=w768) -> (x != y?=w767:bool)
    n481 = case shown="真" w767 {
      tunnel: [w773 w777] -> w771
      tunnel: w764 -> [_ w776]
      tunnel: w766 -> [w773 w775]
      frame False {
      }
      frame True {
        # "文件发生改变进行更新"
        n482 = call <vilib>:"Open Config Data.vi"("error in (no error)"=w775, "configuration file path"=w776) -> ("error out"=w781:errorcluster, "refnum"=w780:T12)  [unwired: 7 in, 1 out]
        n483 = vi-ref "总氮断电保存全局变量.vi"() -> (w774:refnum<vi>)
        n484 = call <userlib>:"Read Panel from INI__ogtk.vi"("error in (no error)"=w781, "VI ref"=w774, "refnum"=w780) -> ("error out"=w779:errorcluster, "refnum out"=w778:T12)  [unwired: 7 in]
        n485 = call <vilib>:"Close Config Data.vi"("error in (no error)"=w779, "refnum"=w778) -> ("error out"=w777:errorcluster)  [unwired: 8 in, 1 out]
      }
    }
    n486 = Wait (ms)(milliseconds to wait=u32 1000 ("等待时间（毫秒）")) -> ()  [unwired: 1 out]
  }
